vi "WSVCAP SHL FPGA TL Top Level.vi"() -> ()   [LabVIEW 2017]
uses:
  Type Defs/WSVCAP SHL State.ctl
  Type Defs/WSVCAP SHL Transaction Enum.ctl
  Type Defs/WSVCAP SHL Communication Loop State.ctl
  Type Defs/WSVCAP SHL FIFO Operation Enum.ctl
  Type Defs/WSVCAP SHL Operation Step Enum.ctl
  Type Defs/WSVCAP SHL Procedure Step Enum.ctl
  Type Defs/WSVCAP SHL Transaction Step Enum.ctl
  user.lib/Utilities/Type Defs/MISC IO Choice Enum.ctl
  <vilib>/Platform/TimedLoop/XDataNode/timing_clust.ctl
  <vilib>/Platform/TimedLoop/XDataNode/nitl_modes.ctl
  <vilib>/Platform/TimedLoop/XDataNode/wakeup.ctl
  <vilib>/rvi/Emulation/niFpgaGetClockAttributes.vi
  <vilib>/rvi/Emulation/niFpgaSctlEmulationGetInTimedLoop.vi
  <vilib>/rvi/Emulation/niFpgaEmulationReportErrorSimple.vi
  <vilib>/rvi/Emulation/niFpgaProcessEmulError.vi
  <vilib>/rvi/Emulation/niFpgaCriticalErrorInLSC.vi
  <vilib>/Platform/TimedLoop/XDataNode/XDataNode.xnode
  WSVCAP Shell FPGA Low Level/WSVCAP SHL FPGA LL I2C Debug Global.vi
  <vilib>/Platform/TimedLoop/XDataNode/XDNodeRunTimeDep.lvlib
  WSVCAP Shell FPGA Low Level/WSVCAP SHL FPGA LL RFFE Debug Global.vi
  WSVCAP Shell FPGA Low Level/FPGA-SRL/FPGA-SRL.lvlib
  WSVCAP Shell FPGA Low Level/FPGA-SRL/Debug Global.vi
panel:
  in  "UUT Set":u8=8
  in  "Stop Cycle":bool
  out "Cycle Count":u64
  in  "Socket Mask":u32=1 format="%06x"
  out "Display CH (1-48)":i32=1 min=1 max=48 step=1
  out "Status":i32
  out "Read Data":u64
  in  "Transaction":T1
  in  "Bytes to Write":u8=8
  in  "Sub Address":u8=1 format="%02x"
  in  "Ack Read Status":bool
  out "Read Status Flag":bool
  in  "Exit":bool
  out "Waveform Chart":cluster{i16, i16, i16, i16}(graph)
  in  "Wait Ticks":u32=20
  in  "Slave Address":u8=1 format="%02x"
  in  "Bytes to Read":u8=8
  in  "Start":bool
  in  "Cmd":T2
  in  "Ack Read":bool
  out "Read Flag":bool
  in  "Write Flag":bool
  in  "Write Data":u64
  # "Control"
  # "Configuration Parameters"
  # "Host Data Transfer"
  # "Command Type"
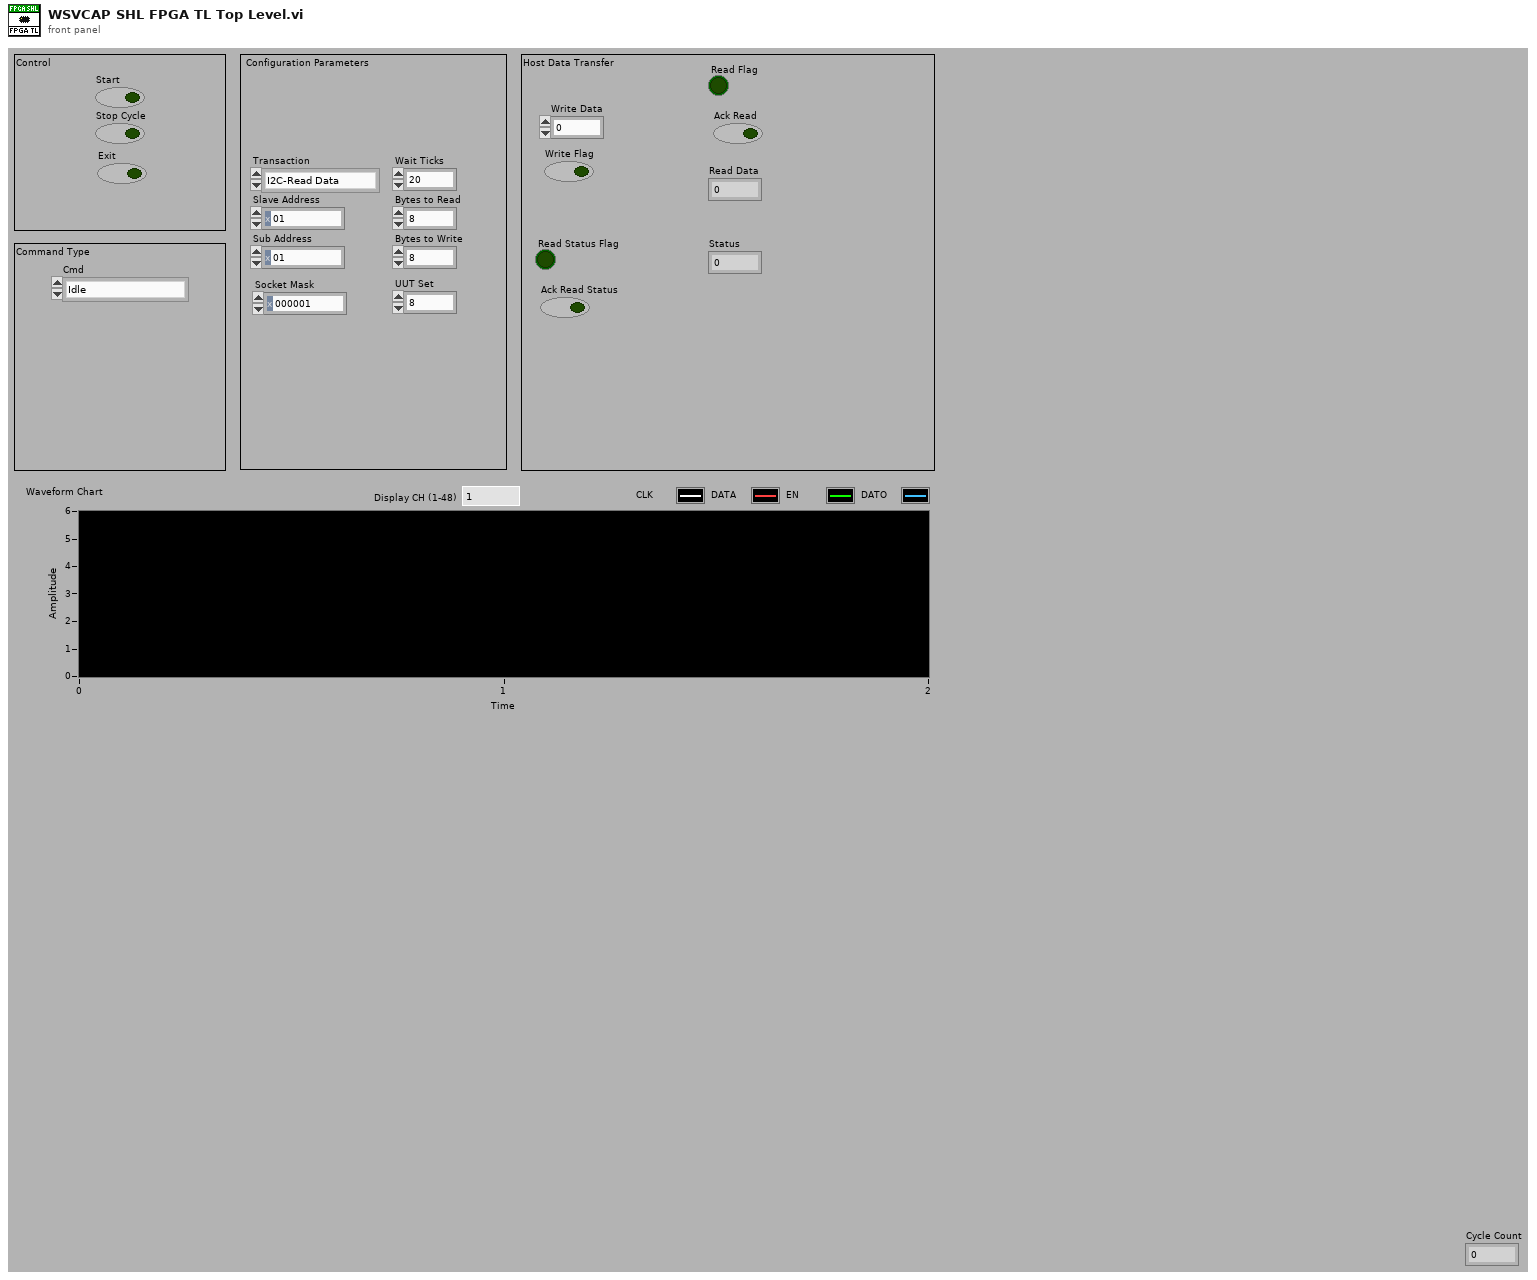
[diagram p1: front panel]
types:
  T1 = typedef "WSVCAP SHL Transaction Enum.ctl" = enum16{"I2C-Read Data", "I2C-Write Data", "RFFE-Ext Write", "RFFE-Ext Read", "SRL-Write Data"}
  T2 = typedef "WSVCAP SHL State.ctl" = enum8{"Idle", "Transfer Data"}
  T3 = typedef "WSVCAP SHL Communication Loop State.ctl" = enum8{"Idle", "Initialize", "Pre-Transmission", "Transmit Data", "Post Transmition", "Operation Complete"}
  T4 = typedef "WSVCAP SHL FIFO Operation Enum.ctl" = enum16{"Create FIFO/Memory", "Get Write FIFO Status", "Get Read FIFO Status", "Put Element in Write", "Put Element in Read", "Get Element from Write", "Get Element from Read"}
  T5 = typedef "WSVCAP SHL Procedure Step Enum.ctl" = enum16{"I2C Start/Stop - 1: Set Clock Low", "I2C Start/Stop - 2: Wait", "I2C Start/Stop - 3: Set Data I", "I2C Start/Stop - 4: Wait", "I2C Start/Stop - 5: Set Clock High", "I2C Start/Stop - 6: Wait", "I2C Start/Stop - 7: Set Data II", "I2C Start/Stop - 8: Wait", "I2C Start/Stop - 9: Set Clock Low", "I2C Start/Stop - 10: Wait", "I2C Read ACK - 1: Set Clock High", "I2C Read ACK - 2: Wait", "I2C Read ACK - 3: Read ACK Bit", "I2C Read ACK - 4: Wait", "I2C Read ACK - 5: Set Clock Low", "I2C Read ACK - 6: Wait", "I2C Write ACK - 1: Write ACK Bit", "I2C Write ACK - 2: Wait", "I2C Write ACK - 3: Set Clock High", "I2C Write ACK - 4: Wait", "I2C Write ACK - 5: Set Clock Low", "I2C Write ACK - 6: Wait", "I2C Write ACK - 7: Set Data Low", "I2C Send Add - 1: Reset Bits Remaining", "I2C Send Add - 2: Set Data Bit", "I2C Send Add - 3: Wait", "I2C Send Add - 4: Set Clock High", "I2C Send Add - 5: Wait", "I2C Send Add - 6: Set Clock Low", "I2C Send Add - 7: Wait", "I2C Send Add - 8: Check Bits Remaining", "I2C Send Data - 1: Reset Bits Remaining", "I2C Send Data - 2: Load Write Bit from FIFO", "I2C Send Data - 3: Set Data Bit", "I2C Send Data - 4: Wait", "I2C Send Data - 5: Set Clock High", "I2C Send Data - 6: Wait", "I2C Send Data - 7: Set Clock Low", "I2C Send Data - 8: Wait", "I2C Send Data - 9: Check Bits Remaining", "I2C Receive Data - 1: Reset Bits Remaining", "I2C Receive Data - 2: Wait", "I2C Receive Data - 3: Set Clock High", "I2C Receive Data - 4: Wait", "I2C Receive Data - 5: Read Data Bit", "I2C Receive Data - 6: Wait", "I2C Receive Data - 7: Set Clock Low", "I2C Receive Data - 8: Wait", "I2C Receive Data - 9: Check Bits Remaining", "RFFE Send SSC - 1:Set Low", "RFFE Send SSC - 2:Wait", "RFFE Send SSC - 3:Set SDA High", "RFFE Send SSC - 4:Wait", "RFFE Send SSC - 5:Set SDA Low", "RFFE Send SSC - 6:Wait", "RFFE Send Data - 1:Set SCL High", "RFFE Send Data - 2:Wait", "RFFE Send Data - 3:Set SCL Low", "RFFE Send Data - 4:Wait", "RFFE Send Data - 5:Set SCL High (P)", "RFFE Send Data - 6:Wait", "RFFE Send Data - 7:Set SCL Low (P)", "RFFE Send Data - 8:Wait", "RFFE Send Data - 9:Set SCL High (BP)", "RFFE Send Data - 10:Wait", "RFFE Send Data - 11:Set SCL Low (BP)", "RFFE Send Data - 12:Wait", "RFFE Receive Data - 1:Set SCL High", "RFFE Receive Data - 2:Wait", "RFFE Receive Data - 3:Set SCL Low", "RFFE Receive Data - 4:Wait", "RFFE Receive Data - 5:Set SCL High (BP)", "RFFE Receive Data - 6:Wait", "RFFE Receive Data - 7:Set SCL Low (BP)", "RFFE Receive Data - 8:Wait", "RFFE Wait CMD Delay - 1:Wait", "RFFE Clear Lines - 1:Clear", "SRL Write Data - 1:Set SYNC High", "SRL Write Data - 2:Wait SYNC Delay", "SRL Write Data - 3:Set SYNC Low", "SRL Write Data - 4:Set SCLK High", "SRL Write Data - 5:Wait", "SRL Write Data - 6:Set SCLK Low", "SRL Write Data - 7:Wait", "SRL Write Data - 8:Set SYNC High", "SRL Wait CMD Delay - 1:Wait", "SRL Clear Lines - 1:Clear"}
  T6 = typedef "WSVCAP SHL Operation Step Enum.ctl" = enum16{"I2C Send Slave Add - A: Send Start Sequence", "I2C Send Slave Add - B: Load Address Byte", "I2C Send Slave Add - C: Send Address Byte", "I2C Send Slave Add - D: Read Slave ACK", "I2C Send Sub Add - A: Load Sub Address", "I2C Send Sub Add - B: Send Address Byte", "I2C Send Sub Add - C: Read Slave ACK", "I2C Send Data - A: Get Byte from FIFO", "I2C Send Data - B: Send Data Byte", "I2C Send Data - C: Read Slave ACK", "I2C Send Data - D: Send Stop Sequence", "I2C Read Data - A: Load Bytes to Read", "I2C Read Data - B: Receive Byte", "I2C Read Data - C: Write Master ACK", "I2C Read Data - D: Send Stop Sequence", "RFFE Read Data - A: Send SSC", "RFFE Read Data - B: Send CMD Frame", "RFFE Read Data - C: Receive Byte", "RFFE Write Data - A: Send SSC", "RFFE Write Data - B: Send Data", "RFFE Write Data - C: Wait CMD Delay", "RFFE Write Data - D: Clear Lines", "SRL Write Data - A: Send Data", "SRL Write Data - B: Wait CMD Delay", "SRL Write Data - C: Clear Lines"}
  T7 = typedef "WSVCAP SHL Transaction Step Enum.ctl" = enum16{"I2C Write - I:Send Slave Address", "I2C Write - II:Send Sub Address", "I2C Write - III:Send Data Bytes", "I2C Read - I:Send Slave Address (W)", "I2C Read - II:Send Sub Address", "I2C Read - III:Send Slave Address (R)", "I2C Read - IV:Read Data Bytes", "RFFE Ext Write - I.Write Data", "RFFE Ext Read - I:Read Data", "SRL Write - I:Write Data"}
  T8 = typedef "MISC IO Choice Enum.ctl" = enum16{"Read", "Write"}
  T9 = typedef "XDNodeRunTimeDep.lvlib/timing_clust.ctl" = cluster{"Expected End [f-1]":u64, "Actual End [f-1]":u64, "Finished Late? [f-1]":bool, "Expected End [i-1]":u64, "Actual End [i-1]":u64, "Finished Late? [i-1]":bool, "Expected Start [i]":u64, "Actual Start [i]":u64, "Expected Start [f]":u64, "Actual Start [f]":u64, "Source Name":string, "Structure Name":string, "Period":i64, "Deadline":i64, "Offset":i64, "Start":i64, "Priority":i32, "Timeout":i32, "Mode":T10, "Wakeup Reason":T11, "Error":errorcluster, "Source Type":string, "Secondary Source Type":string, "Global End Time":u64, "Global Start Time":u64, "Frame Duration":u64, "Iteration Duration":u64, "Assigned CPU":i32, "I/O Scan Engine Mode":u32}
  T10 = typedef "XDNodeRunTimeDep.lvlib/nitl_modes.ctl" = enum32{"No Change", "Process missed periods, maintain original phase", "Discard missed periods, maintain original phase", "Process missed periods, ignore original phase", "Discard missed periods, ignore original phase"}
  T11 = typedef "XDNodeRunTimeDep.lvlib/wakeup.ctl" = enum32{"Normal", "Aborted", "Asynchronous wakeup", "Timing source error", "Timed loop error", "Timeout"}
  T12 = typedef "WSVCAP SHL Transaction Cluster.ctl" = cluster{"Transaction":T1, "Write Byte":u8, "Write Bits Remaining":u8, "Read Bits Remaining":u8, "Read Bytes Remaining":u8, "Wait Ticks Remaining":u32, "Slave Address":u8, "Bytes to Read":u8, "Bytes to Write":u8, "Sub Address":u8, "Socket Mask":u32, "Write CMD Idx [0-95]":u8, "Write Bit Index [0-18]":u8, "CMD Delay (Ticks)":u32, "Commands per Cycle [1-96]":u8, "CMD Length [1-48]":u8, "Cycle Count":u64, "Cycle Mode":bool, "Cycle CMD":u64, "Transaction Step":T7, "Operation Step":T6, "Procedure Step":T5, "Start Operation":bool, "Start Procedure":bool, "Procedure":T13, "Wait Ticks":u32, "UUT Set (0/1)":u8}
  T13 = typedef "WSVCAP SHL Procedure Enum.ctl" = enum16{"None", "I2C-Send Start/Stop Sequence", "I2C-Send Address Byte", "I2C-Send Data Byte", "I2C-Read ACK", "I2C-Receive Byte", "I2C-Write ACK", "RFFE-Clear Lines", "RFFE-Send SSC", "RFFE-Send Data", "RFFE-Receive Data", "RFFE-Wait CMD Delay", "SRL-Clear Lines", "SRL-Send Data", "SRL-Wait CMD Delay"}
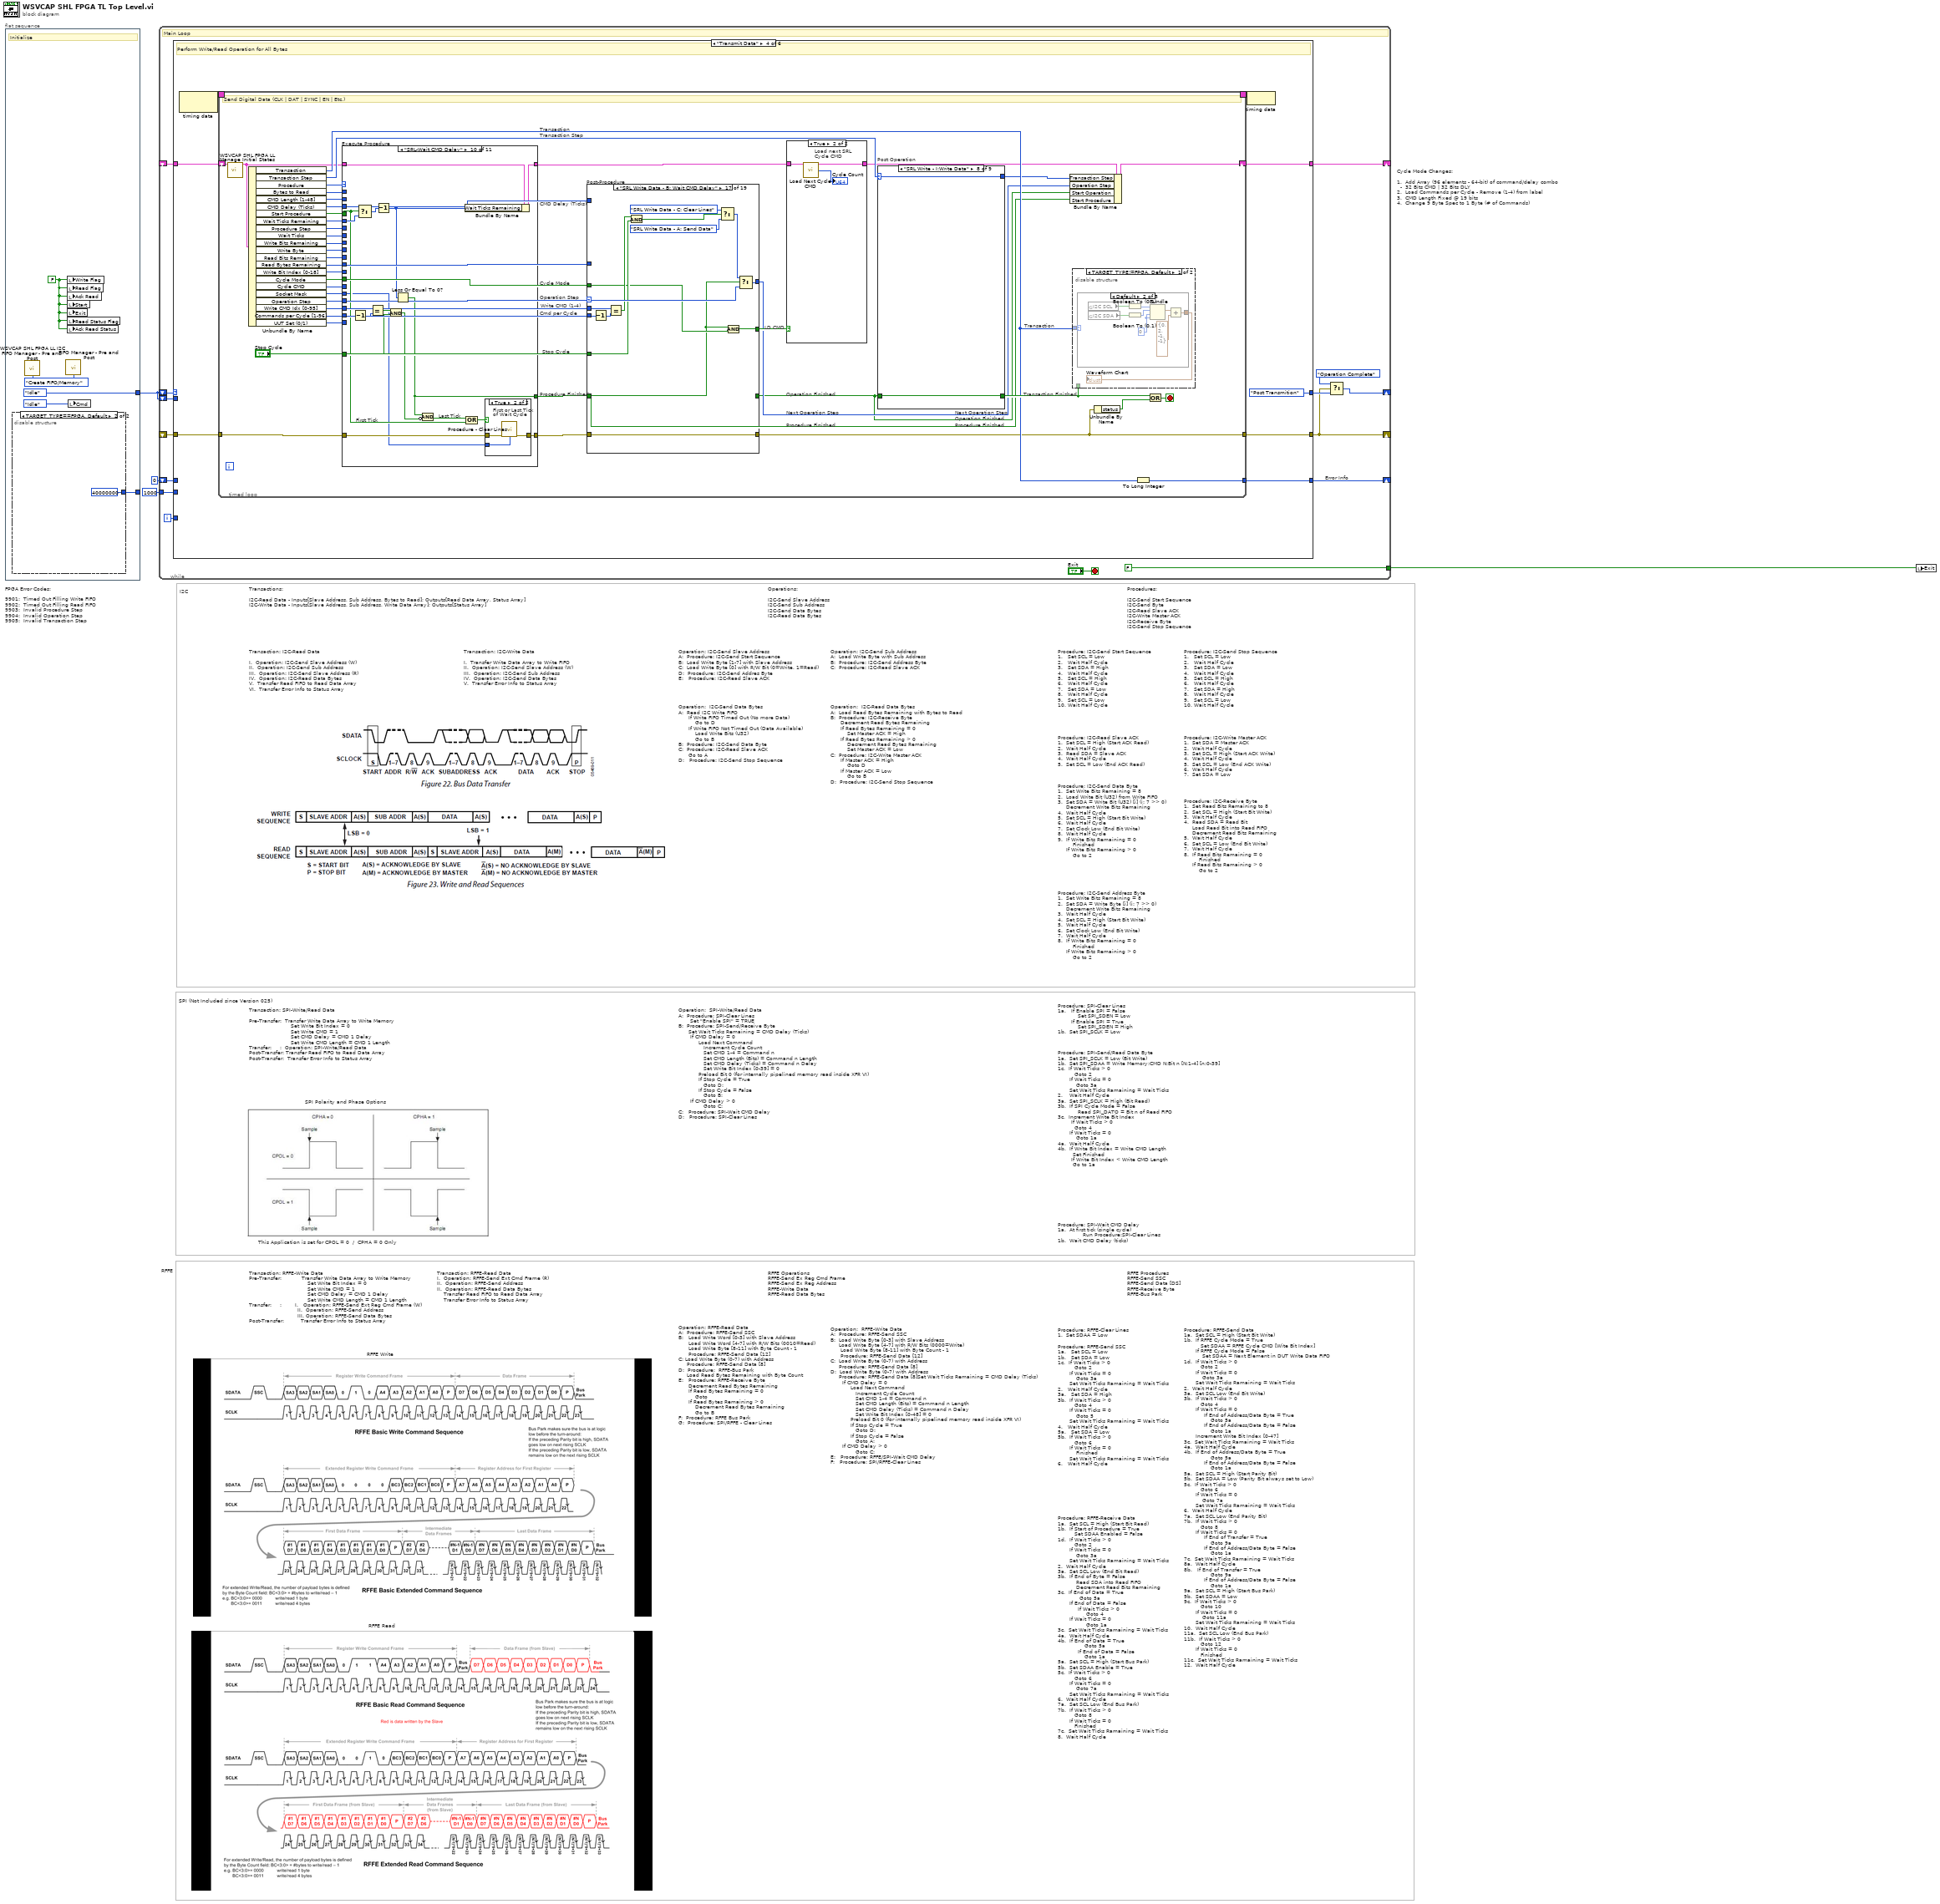
[diagram p0: block diagram]
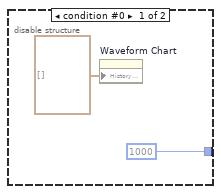
[diagram p2: hidden frame]
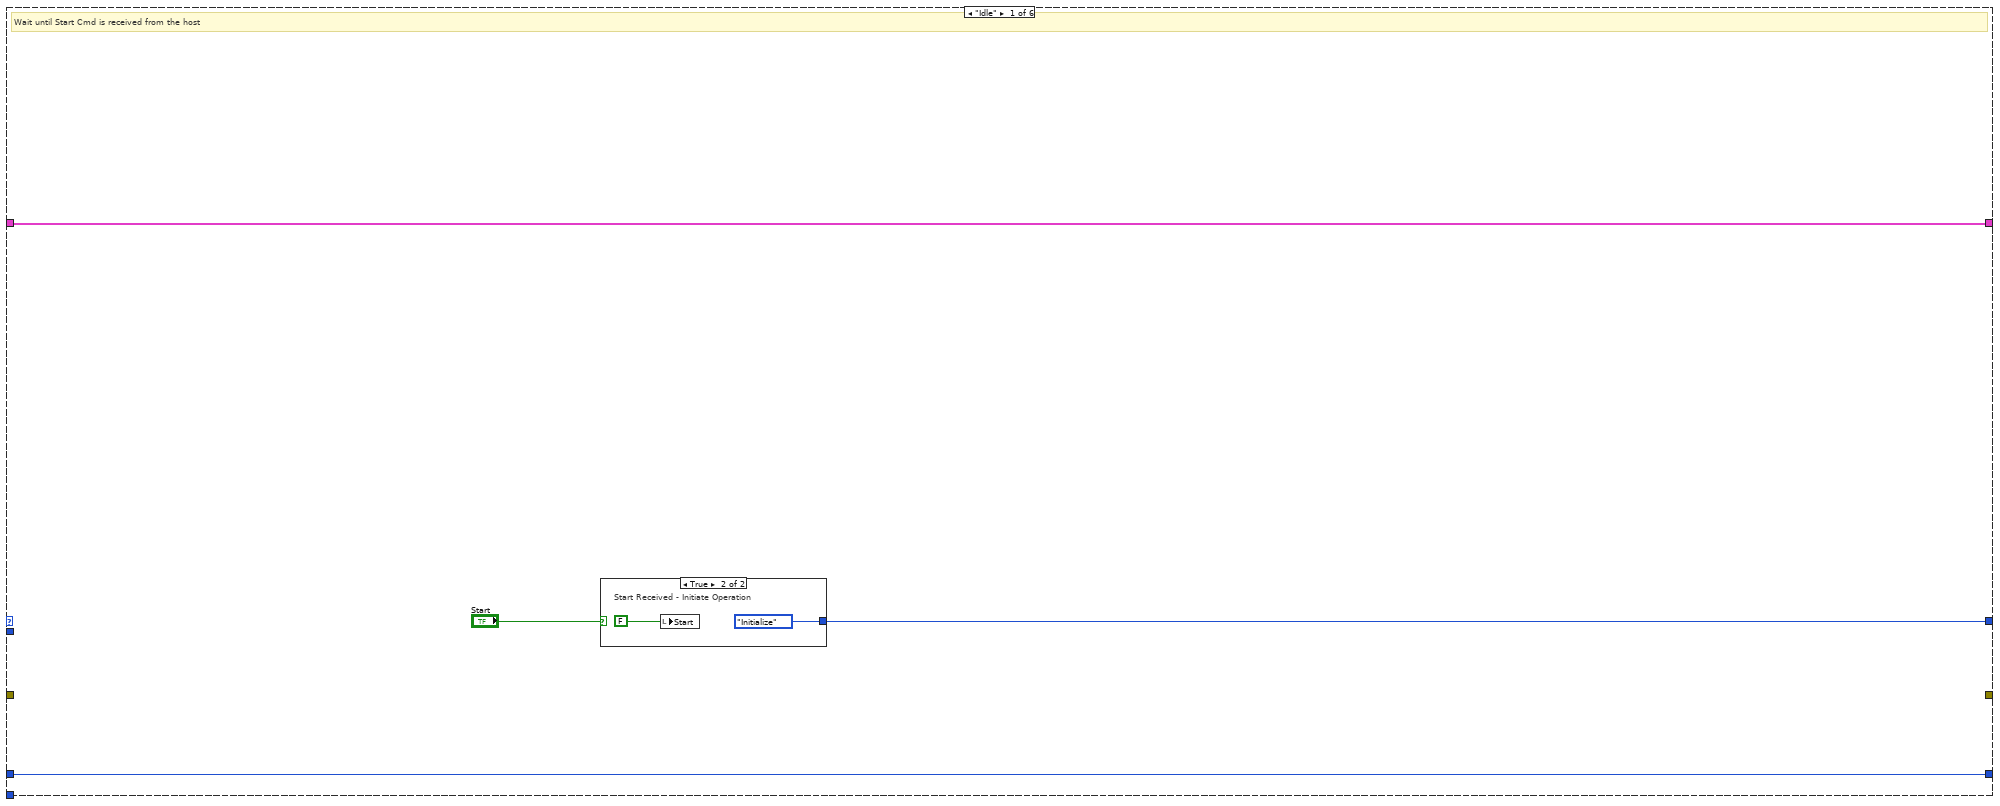
[diagram p3: hidden frame]
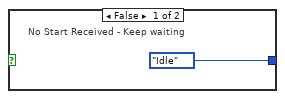
[diagram p4: hidden frame]
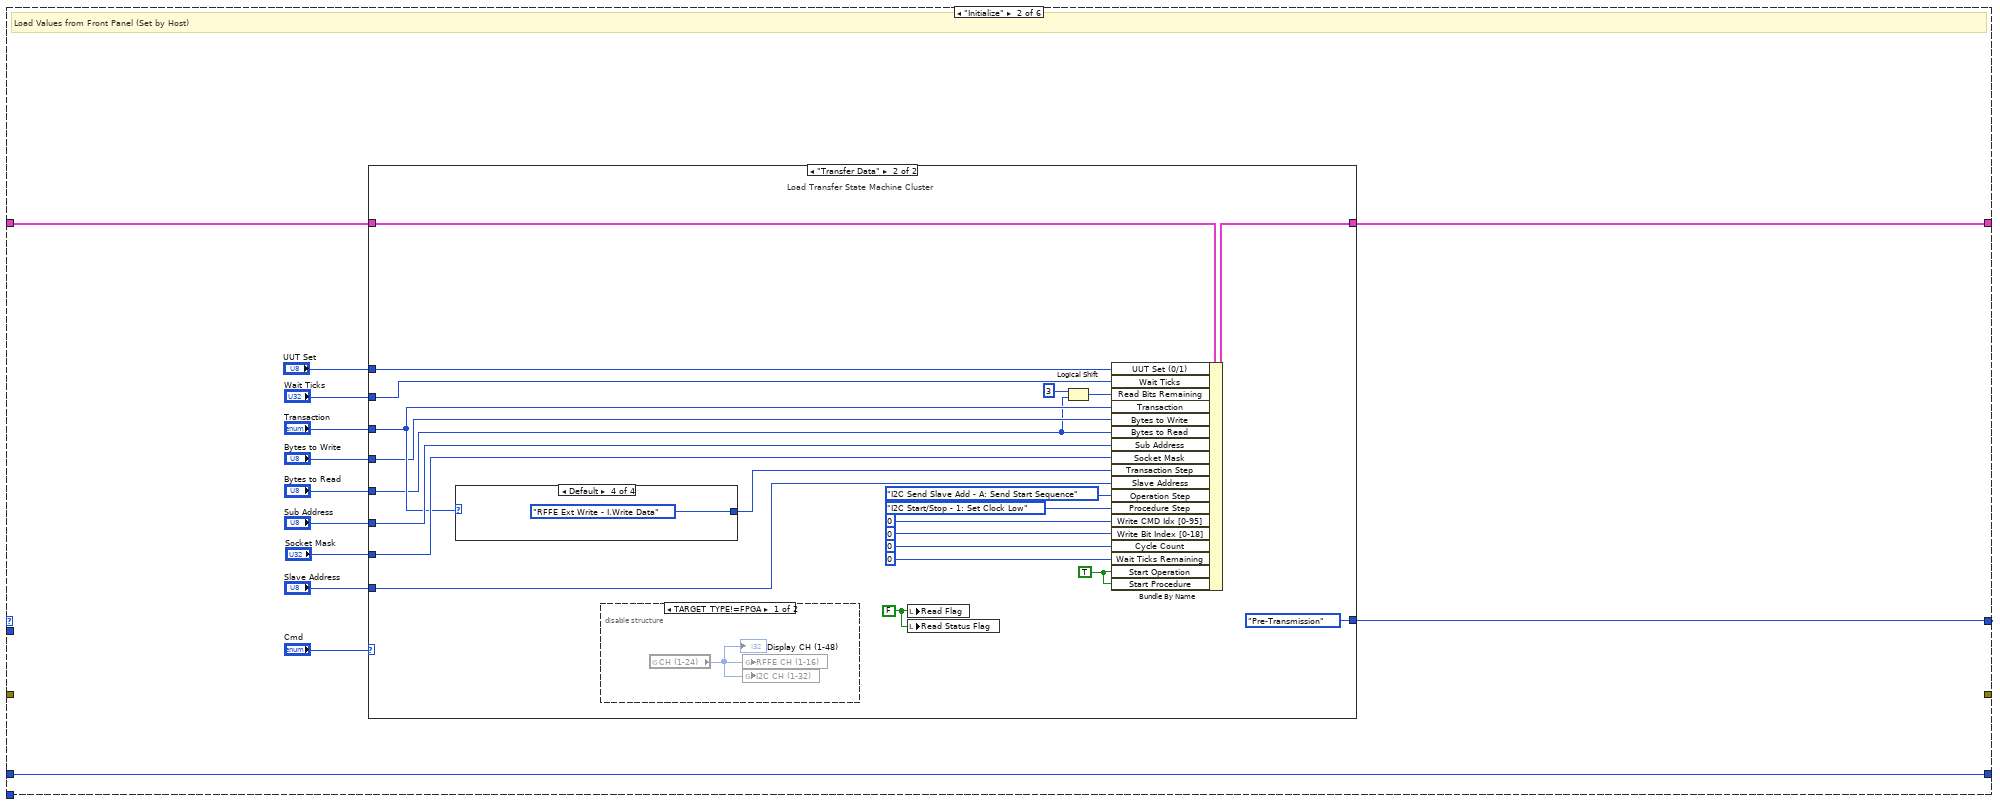
[diagram p5: hidden frame]
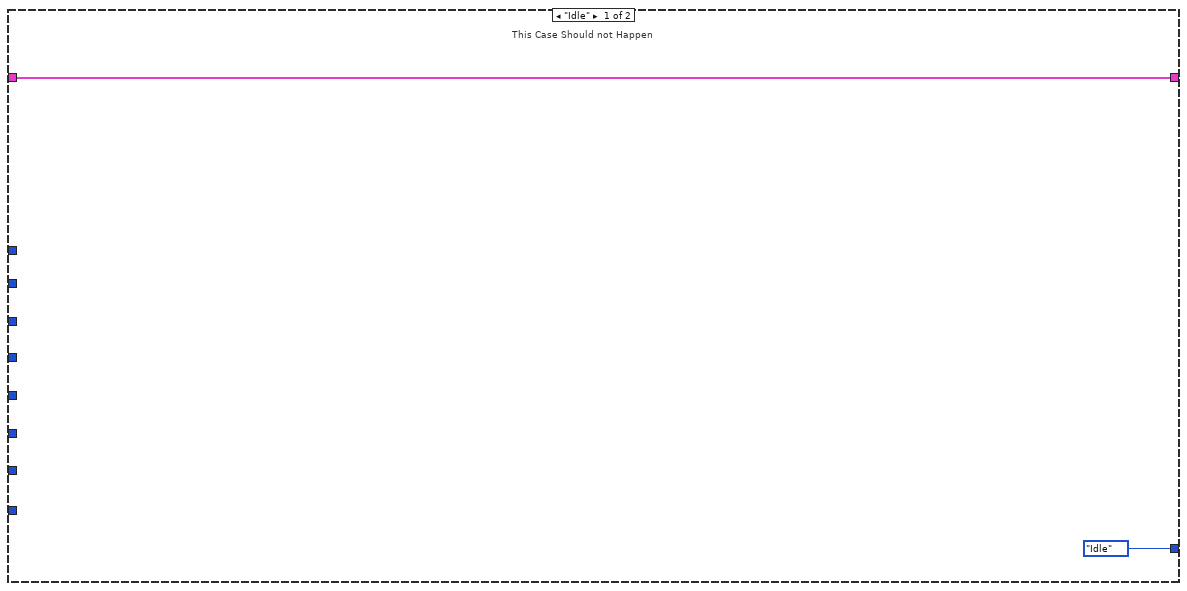
[diagram p6: hidden frame]
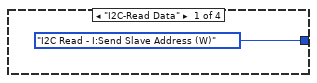
[diagram p7: hidden frame]
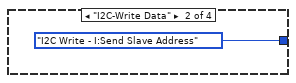
[diagram p8: hidden frame]
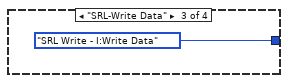
[diagram p9: hidden frame]
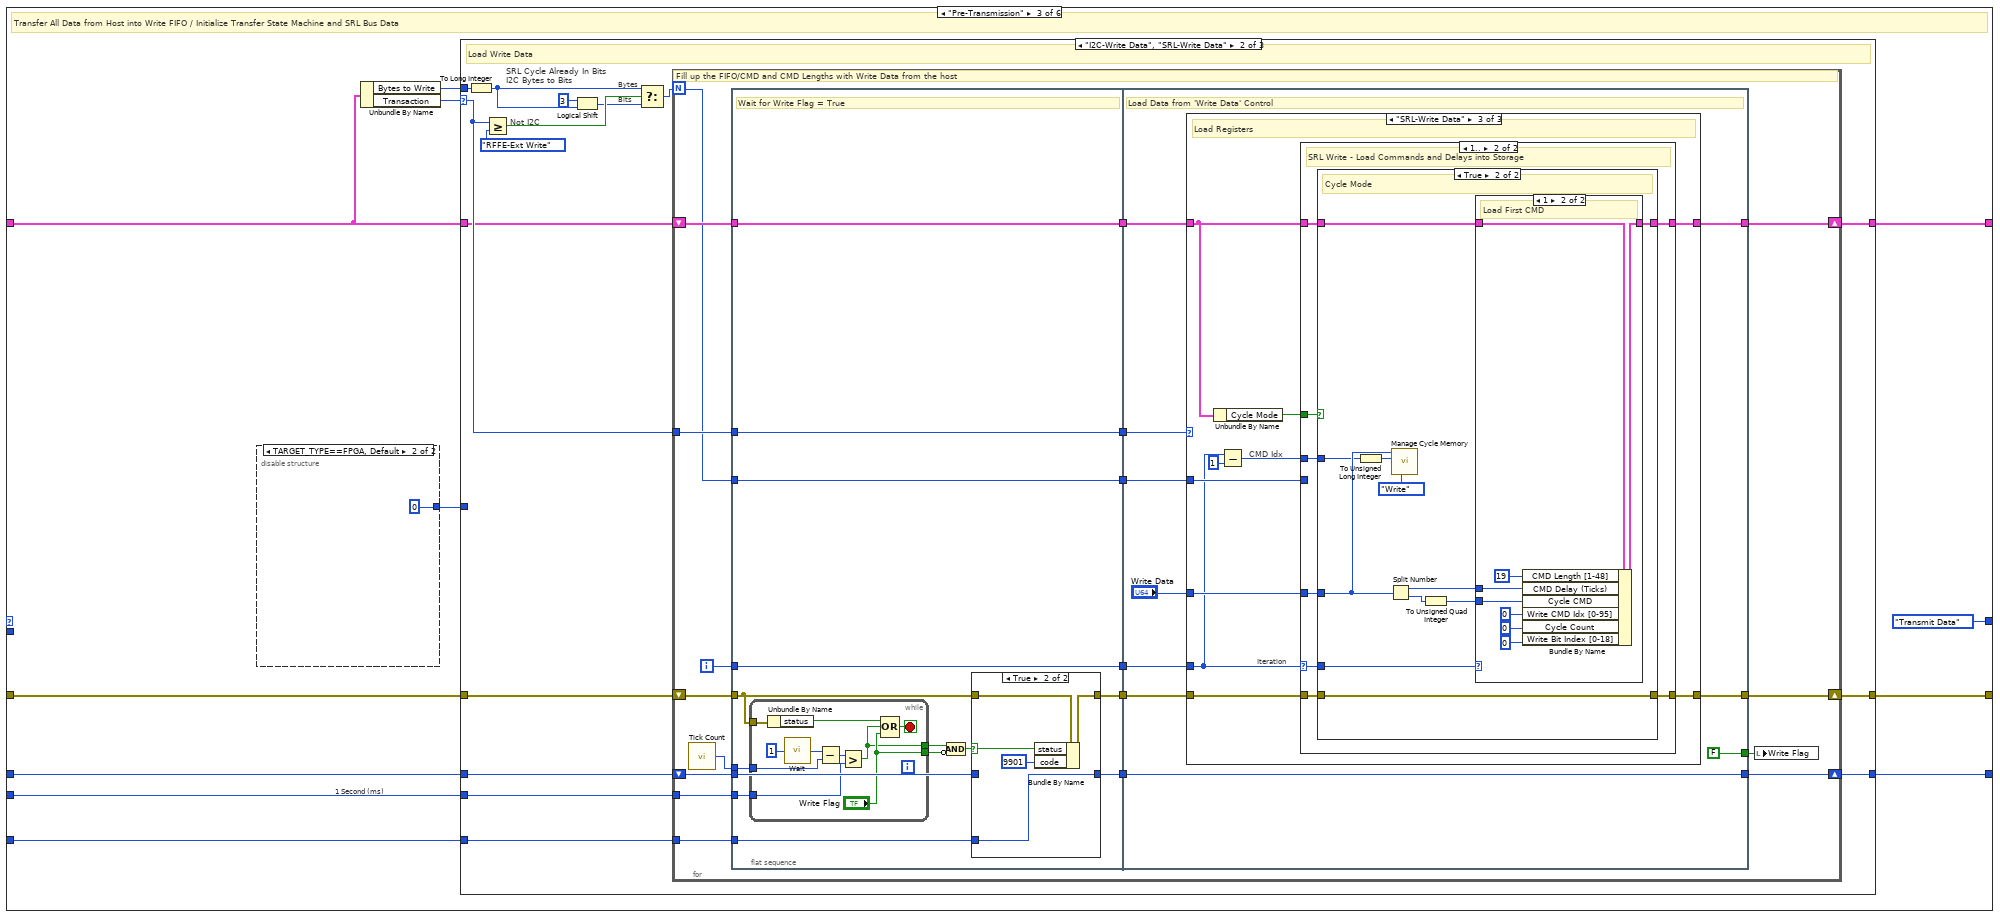
[diagram p11: hidden frame]
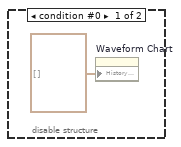
[diagram p12: hidden frame]
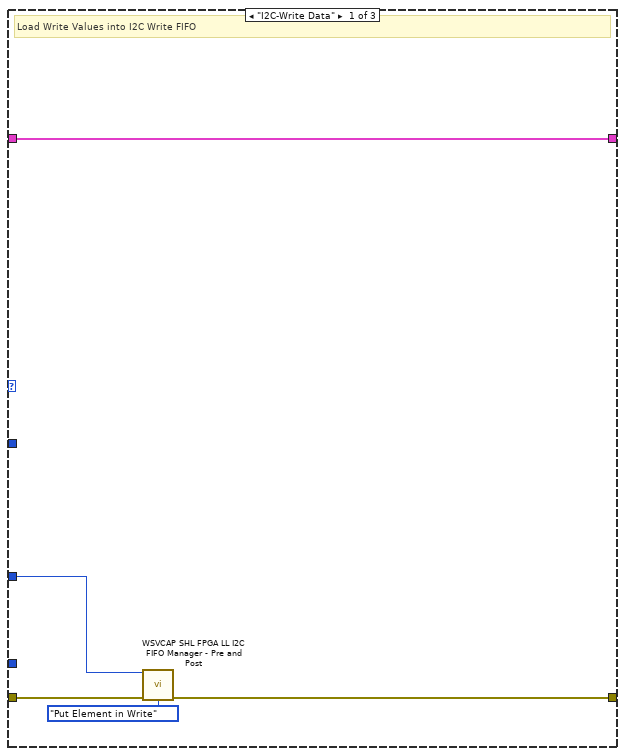
[diagram p15: hidden frame]
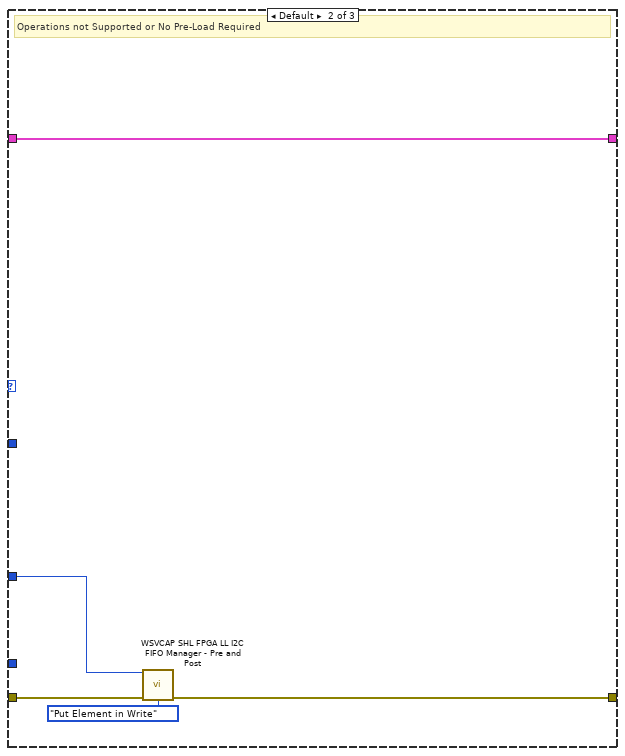
[diagram p16: hidden frame]
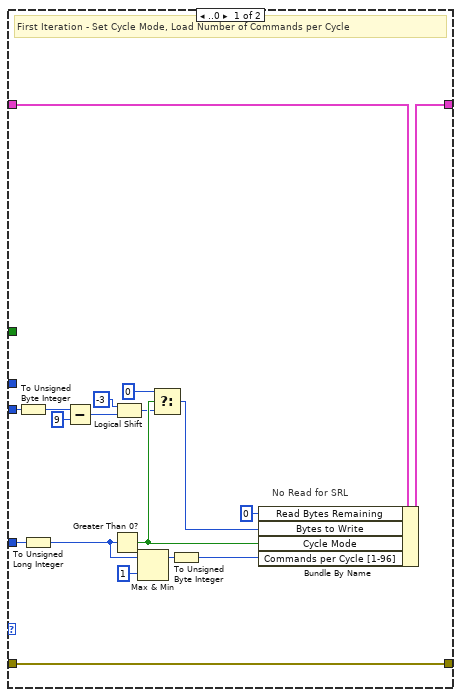
[diagram p17: hidden frame]
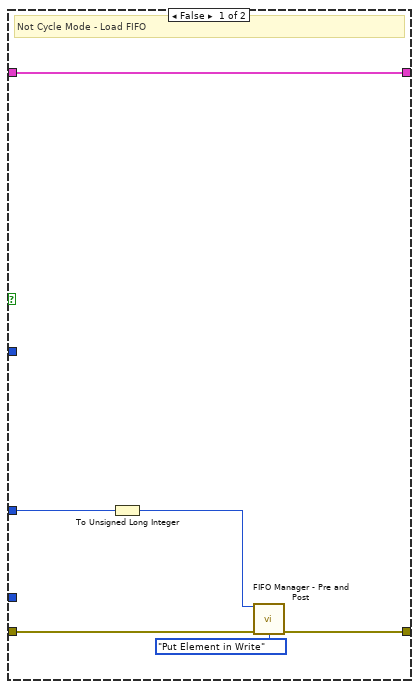
[diagram p18: hidden frame]
diagram:
  # "Cycle Mode Changes:\n\n1.  Add Array (96 elements - 64-bit) of command/delay combo\n  -  32 Bits CMD | 32 Bits DLY\n2.  Load Commands per Cycle - Remove (1-4) from label\n3.  CMD Length Fixed @ 19 bits\n4.  Change 9 Byte Spec to 1 Byte (# of Commands)"
  # "RFFE"
  # "SPI (Not Included since Version 025)"
  # "I2C"
  # "Procedure: RFFE-Receive Data\n1a.  Set SCL = High (Start Bit Read)\n1b.  If Start of Procedure = True\n          Set SDAA Enabled = False\n1d.  If Wait Ticks > 0\n          Goto 2\n       If Wait Ticks = 0 \n           Goto 3a\n       Set Wait Ticks Ramaining = Wait Ticks\n2.  Wait Half Cycle\n3a.  Set SCL Low (End Bit Read)\n3b.  If End of Byte = False\n           Read SDA into Read FIFO\n           Decrement Read Bits Remaining\n3c.  If End of Data = True\n             Goto 5a\n       If End of Data = False\n            If Wait Ticks > 0\n                 Goto 4\n       If Wait Ticks = 0         \n                 Goto 1a\n3c.  Set Wait Ticks Ramaining = Wait Ticks     \n4a.  Wait Half Cycle\n4b.  If End of Data = True\n                Goto 5a\n            If End of Data = False\n                Goto 1a\n5a.  Set SCL = High (Start Bus Park)\n5b.  Set SDAA Enable = True\n5c.  If Wait Ticks > 0\n          Goto 6\n       If Wait Ticks = 0 \n           Goto 7a\n       Set Wait Ticks Ramaining = Wait Ticks\n6.  Wait Half Cycle\n7a.  Set SCL Low (End Bus Park)\n7b.  If Wait Ticks > 0\n          Goto 8\n       If Wait Ticks = 0 \n          Finished\n7c.  Set Wait Ticks Ramaining = Wait Ticks\n8.  Wait Half Cycle"
  # "Procedure: RFFE-Send Data\n1a.  Set SCL = High (Start Bit Write)\n1b.  If RFFE Cycle Mode = True\n          Set SDAA = RFFE Cycle CMD [Wite Bit Index]\n       If RFFE Cycle Mode = False\n           Set SDAA = Next Element in DUT Write Data FIFO\n1d.  If Wait Ticks > 0\n          Goto 2\n       If Wait Ticks = 0 \n           Goto 3a\n       Set Wait Ticks Ramaining = Wait Ticks\n2.  Wait Half Cycle\n3a.  Set SCL Low (End Bit Write)\n3b.  If Wait Ticks > 0\n          Goto 4\n       If Wait Ticks = 0 \n            If End of Address/Data Byte = True\n                Goto 5a\n            If End of Address/Data Byte = False\n                Goto 1a\n       Increment Write Bit Index [0-47]\n3c.  Set Wait Ticks Ramaining = Wait Ticks     \n4a.  Wait Half Cycle\n4b.  If End of Address/Data Byte = True\n                Goto 5a\n            If End of Address/Data Byte = False\n                Goto 1a\n5a.  Set SCL = High (Start Parity Bit)\n5b.  Set SDAA = Low (Parity Bit always set to Low)\n5c.  If Wait Ticks > 0\n          Goto 6\n       If Wait Ticks = 0 \n           Goto 7a\n       Set Wait Ticks Ramaining = Wait Ticks\n6.  Wait Half Cycle\n7a.  Set SCL Low (End Parity Bit)\n7b.  If Wait Ticks > 0\n          Goto 8\n       If Wait Ticks = 0 \n            If End of Transfer = True\n                Goto 9a\n            If End of Address/Data Byte = False\n                Goto 1a\n7c.  Set Wait Ticks Ramaining = Wait Ticks\n8a.  Wait Half Cycle\n8b.   If End of Transfer = True\n                Goto 9a\n            If End of Address/Data Byte = False\n                Goto 1a\n9a.  Set SCL = High (Start Bus Park)\n9b.  Set SDAA = Low\n9c.  If Wait Ticks > 0\n          Goto 10\n       If Wait Ticks = 0 \n           Goto 11a\n       Set Wait Ticks Ramaining = Wait Ticks\n10.  Wait Half Cycle\n11a.  Set SCL Low (End Bus Park)\n11b.  If Wait Ticks > 0\n          Goto 12\n       If Wait Ticks = 0 \n          Finished\n11c.  Set Wait Ticks Ramaining = Wait Ticks\n12.  Wait Half Cycle"
  # "Procedure: RFFE-Send SSC\n1a.   Set SCL = Low\n1b.   Set SDA = Low\n1c.  If Wait Ticks > 0\n          Goto 2\n       If Wait Ticks = 0 \n           Goto 3a\n       Set Wait Ticks Ramaining = Wait Ticks\n2.   Wait Half Cycle\n3a.   Set SDA = High\n3b.  If Wait Ticks > 0\n          Goto 4\n       If Wait Ticks = 0 \n           Goto 5\n       Set Wait Ticks Ramaining = Wait Ticks\n4.   Wait Half Cycle\n5a.   Set SDA = Low\n5b.  If Wait Ticks > 0\n          Goto 6\n       If Wait Ticks = 0 \n           Finished\n       Set Wait Ticks Ramaining = Wait Ticks\n6.   Wait Half Cycle"
  # "Procedure: SPI-Clear Lines\n1a.   If Enable SPI = False\n            Set SPI_SDEN = Low\n        If Enable SPI = True\n            Set SPI_SDEN = High\n1b.  Set SPI_SCLK = Low"
  # "Procedure: RFFE-Clear Lines\n1.  Set SDAA = Low"
  # "Operation:  RFFE-Write Data\nA:  Procedure: RFFE-Send SSC\nB:  Load Write Byte [0-3] with Slave Address\n     Load Write Byte [4-7] with R/W Bits (0000=Write)\n      Load Write Byte [8-11] with Byte Count - 1\n      Procedure: RFFE-Send Data [12]\nC:  Load Write Byte (0-7) with Address\n     Procedure: RFFE-Send Data [8]\nD:  Load Write Byte (0-7) with Address\n     Procedure: RFFE-Send Data [8]Set Wait Ticks Remaining = CMD Delay (Ticks)\n       If CMD Delay = 0\n            Load Next Command\n               Increment Cycle Count\n               Set CMD 1-4 = Command n\n               Set CMD Length (Bits) = Command n Length\n               Set CMD Delay (Ticks) = Command n Delay\n               Set Write Bit Index [0-48] = 0\n            Preload Bit 0 (for internally pipelined memory read inside XFR VI)\n            If Stop Cycle = True\n               Goto D:\n            If Stop Cycle = False\n               Goto A:\n       If CMD Delay > 0\n               Goto C:\nE:   Procedure: RFFE/SPI-Wait CMD Delay          \nF:   Procedure: SPI/RFFE-Clear Lines"
  # "Operation: RFFE-Read Data\nA:  Procedure: RFFE-Send SSC\nB:   Load Write Word [0-3] with Slave Address\n      Load Write Word [4-7] with R/W Bits (0010=Read)\n      Load Write Byte [8-11] with Byte Count - 1\n      Procedure: RFFE-Send Data [12]\nC: Load Write Byte (0-7) with Address\n     Procedure: RFFE-Send Data [8]\nD:  Procedure:  RFFE-Bus Park\n     Load Read Bytes Remaining with Byte Count\nE:   Procedure: RFFE-Receive Byte\n      Decrement Read Bytes Remaining\n      If Read Bytes Remaining = 0\n          Goto\n      If Read Bytes Remaining > 0\n          Decrement Read Bytes Remaining\n          Go to B\nF:  Procedure: RFFE Bus Park\nG:  Procedure: SPI/RFFE - Clear Lines"
  # "RFFE Write"
  # "RFFE Read"
  # "Transaction: RFFE-Write Data\nPre-Transfer:            Transfer Write Data Array to Write Memory\n                                   Set Write Bit Index = 0\n                                   Set Write CMD = 1\n                                   Set CMD Delay = CMD 1 Delay\n                                   Set Write CMD Length = CMD 1 Length\nTransfer:     :        I.   Operation: RFFE-Send Ext Reg Cmd Frame (W)\n                             II.  Operation: RFFE-Send Address\n                             III. Operation: RFFE-Send Data Bytes\nPost-Transfer:          Transfer Error Info to Status Array"
  # "RFFE Procedures\nRFFE-Send SSC\nRFFE-Send Data [DS]\nRFFE-Receive Byte\nRFFE-Bus Park"
  # "Transaction: RFFE-Read Data\nI.  Operation: RFFE-Send Ext Cmd Frame (R)\nII.  Operation: RFFE-Send Address\nII.  Operation: RFFE-Read Data Bytes\n    Transfer Read FIFO to Read Data Array\n    Transfer Error Info to Status Array"
  # "RFFE Operations\nRFFE-Send Ex Reg Cmd Frame\nRFFE-Send Ex Reg Address\nRFFE-Write Data\nRFFE-Read Data Bytes"
  # "SPI Polarity and Phase Options"
  # "Procedure: SPI-Wait CMD Delay\n1a.  At first tick (single cycle)\n               Run Procedure:SPI-Clear Lines\n1b.  Wait CMD Delay (ticks)"
  # "This Application is set for CPOL = 0  /  CPHA = 0 Only"
  # "Procedure: SPI-Send/Read Data Byte\n1a.  Set SPI_SCLK = Low (Bit Write)\n1b.  Set SPI_SDAA = Write Memory:CMD N:Bit n [N:1-4] [n:0-39] \n1c.  If Wait Ticks > 0\n          Goto 2\n       If Wait Ticks = 0 \n           Goto 3a\n       Set Wait Ticks Ramaining = Wait Ticks\n2.    Wait Half Cycle\n3a.  Set SPI_SCLK = High (Bit Read)\n3b.  If SPI Cycle Mode = False\n            Read SPI_DATO = Bit n of Read FIFO            \n3c.  Increment Write Bit Index\n        If Wait Ticks > 0\n          Goto 4\n       If Wait Ticks = 0 \n           Goto 1a \n4a.  Wait Half Cycle\n4b.  If Write Bit Index = Write CMD Length\n         Set Finished\n        If Write Bit Index < Write CMD Length\n         Go to 1a"
  # "Operation:  SPI-Write/Read Data\nA:  Procedure: SPI-Clear Lines\n       Set \"Enable SPI\" = TRUE \nB:  Procedure: SPI-Send/Receive Byte\n      Set Wait Ticks Remaining = CMD Delay (Ticks)\n       If CMD Delay = 0\n            Load Next Command\n               Increment Cycle Count\n               Set CMD 1-4 = Command n\n               Set CMD Length (Bits) = Command n Length\n               Set CMD Delay (Ticks) = Command n Delay\n               Set Write Bit Index [0-39] = 0\n            Preload Bit 0 (for internally pipelined memory read inside XFR VI)\n            If Stop Cycle = True\n               Goto D:\n            If Stop Cycle = False\n               Goto B:\n       If CMD Delay > 0\n               Goto C:\nC:   Procedure: SPI-Wait CMD Delay          \nD:   Procedure: SPI-Clear Lines"
  # "FPGA Error Codes:\n\n9901:  Timed Out Filling Write FIFO\n9902:  Timed Out Filling Read FIFO\n9903:  Invalid Procedure Step\n9904:  Invalid Operation Step\n9905:  Invalid Transaction Step"
  # "Transaction: SPI-Write/Read Data\n\nPre-Transfer:  Transfer Write Data Array to Write Memory\n                         Set Write Bit Index = 0\n                         Set Write CMD = 1\n                         Set CMD Delay = CMD 1 Delay\n                         Set Write CMD Length = CMD 1 Length\nTransfer:     :  Operation: SPI-Write/Read Data\nPost-Transfer: Transfer Read FIFO to Read Data Array\nPost-Transfer:  Transfer Error Info to Status Array"
  # "Procedure: I2C-Send Address Byte\n1.  Set Write Bits Remaining = 8\n2.  Set SDA = Write Byte [i] (i: 7 >> 0)\n     Decrement Write Bits Remaining\n3.  Wait Half Cycle\n4.  Set SCL = High (Start Bit Write)\n5.  Wait Half Cycle\n6.  Set Clock Low (End Bit Write)\n7.  Wait Half Cycle\n8.  If Write Bits Remaining = 0\n         Finished\n     If Write Bits Remaining > 0\n         Go to 2"
  # "Procedure: I2C-Write Master ACK\n1.  Set SDA = Master ACK\n2.  Wait Half Cycle\n3.  Set SCL = High (Start ACK Write)\n4.  Wait Half Cycle\n5.  Set SCL = Low (End ACK Write)\n6.  Wait Half Cycle\n7.  Set SDA = Low"
  # "Procedure: I2C-Send Start Sequence\n1.   Set SCL = Low\n2.   Wait Half Cycle\n3.   Set SDA = High\n4.   Wait Half Cycle\n5.   Set SCL = High\n6.   Wait Half Cycle\n7.   Set SDA = Low\n8.   Wait Half Cycle\n9.   Set SCL = Low\n10. Wait Half Cycle"
  # "Procedure: I2C-Send Stop Sequence\n1.   Set SCL = Low\n2.   Wait Half Cycle\n3.   Set SDA = Low\n4.   Wait Half Cycle\n5.   Set SCL = High\n6.   Wait Half Cycle\n7.   Set SDA = High\n8.   Wait Half Cycle\n9.   Set SCL = Low\n10. Wait Half Cycle"
  # "Procedure: I2C-Read Slave ACK\n1.  Set SCL = High (Start ACK Read)\n2.  Wait Half Cycle\n3.  Read SDA = Slave ACK\n4.  Wait Half Cycle\n5.  Set SCL = Low (End ACK Read)"
  # "Procedure: I2C-Receive Byte\n1.  Set Read Bits Remaining to 8\n2.  Set SCL = High (Start Bit Write)\n3.  Wait Half Cycle\n4.  Read SDA = Read Bit\n     Load Read Bit into Read FIFO\n     Decrement Read Bits Remaining\n5.  Wait Half Cycle\n6.  Set SCL = Low (End Bit Write)\n7.  Wait Half Cycle\n8.  If Read Bits Remaining = 0\n         Finished\n     If Read Bits Remaining > 0\n         Go to 2"
  # "Procedure: I2C-Send Data Byte\n1.  Set Write Bits Remaining = 8\n2.  Load Write Bit (U32) from Write FIFO\n3.  Set SDA = Write Bit (U32) [i] (i: 7 >> 0)\n     Decrement Write Bits Remaining\n4.  Wait Half Cycle\n5.  Set SCL = High (Start Bit Write)\n6.  Wait Half Cycle\n7.  Set Clock Low (End Bit Write)\n8.  Wait Half Cycle\n9.  If Write Bits Remaining = 0\n         Finished\n     If Write Bits Remaining > 0\n         Go to 2"
  # "Operation:  I2C-Read Data Bytes\nA:  Load Read Bytes Remaining with Bytes to Read\nB:  Procedure: I2C-Receive Byte\n      Decrement Read Bytes Remaining\n      If Read Bytes Remaining = 0\n          Set Master ACK = High\n      If Read Bytes Remaining > 0\n          Decrement Read Bytes Remaining\n          Set Master ACK = Low\nC:  Procedure: I2C-Write Master ACK\n      If Master ACK = High\n          Goto D\n      If Master ACK = Low\n          Go to B\nD:  Procedure: I2C-Send Stop Sequence"
  # "Operation:  I2C-Send Data Bytes\nA:  Read I2C Write FIFO\n      If Write FIFO Timed Out (No more Data)\n          Go to D\n      If Write FIFO Not Timed Out (Data Available)\n          Load Write Bits (U32)\n          Go to B\nB:  Procedure: I2C-Send Data Byte\nC:  Procedure: I2C-Read Slave ACK\n      Go to A\nD:   Procedure: I2C-Send Stop Sequence"
  # "Operation: I2C-Send Sub Address\nA:  Load Write Byte with Sub Address\nB:  Procedure: I2C-Send Address Byte\nC:  Procedure: I2C-Read Slave ACK"
  # "Procedures:\n\nI2C-Send Start Sequence\nI2C-Send Byte\nI2C-Read Slave ACK\nI2C-Write Master ACK\nI2C-Receive Byte\nI2C-Send Stop Sequence"
  # "Transaction: I2C-Write Data\n\nI.  Transfer Write Data Array to Write FIFO\nII.  Operation: I2C-Send Slave Address (W)\nIII.  Operation: I2C-Send Sub Address\nIV.  Operation: I2C-Send Data Bytes\nV.  Transfer Error Info to Status Array"
  # "Transaction: I2C-Read Data\n\nI.  Operation: I2C-Send Slave Address (W)\nII.  Operation: I2C-Send Sub Address\nIII.  Operation: I2C-Send Slave Address (R)\nIV.  Operation: I2C-Read Data Bytes\nV.  Transfer Read FIFO to Read Data Array\nVI.  Transfer Error Info to Status Array"
  # "Transactions:\n\nI2C-Read Data - Inputs[Slave Address, Sub Address, Bytes to Read]; Outputs[Read Data Array, Status Array]\nI2C-Write Data - Inputs[Slave Address, Sub Address, Write Data Array]; Outputs[Status Array]"
  # "Operations:\n\nI2C-Send Slave Address\nI2C-Send Sub Address\nI2C-Send Data Bytes\nI2C-Read Data Bytes"
  # "Operation: I2C-Send Slave Address\nA:  Procedure: I2C-Send Start Sequence\nB:  Load Write Byte [1-7] with Slave Address\nC:  Load Write Byte [0] with R/W Bit (0=Write, 1=Read)\nD:  Procedure: I2C-Send Addres Byte\nE:   Procedure: I2C-Read Slave ACK"
  n1 = flat-sequence {
    tunnel: [WSVCAP_SHL_Communication_Loop_State."Idle" ("Action")] -> w3
    tunnel: [w6] -> _
    frame #0 {
      w5 = WSVCAP_SHL_FIFO_Operation_Enum."Create FIFO/Memory" ("Operation")
      w7 = FALSE ("Done")
      # "Initialize"
      n2 = disable-structure shown="TARGET_TYPE==FPGA, Default" {
        disable-tunnel: [u32 1000 ("x-y") u32 40000000 ("x-y")] -> w6
        frame condition #0 {
          n3 = property on="Waveform Chart" class="WFChart (strict)"("History Data"=cluster{i16, i16, i16, i16}[] []) -> ()  [unwired: 2 in, 2 out]
        }
        frame condition #1 (active) {
        }
      }
      n4 = call "WSVCAP SHL FPGA LL I2C FIFO Manager - Pre and Post.vi"("Operation"=w5) -> ()  [unwired: 12 in, 3 out]
      n5 = call "FIFO Manager - Pre and Post.vi"("Operation"=w5) -> ()  [unwired: 12 in, 3 out]
      n6 = local write "Write Flag"(w7) -> ()
      n7 = local write "Read Flag"(w7) -> ()
      n8 = local write "Ack Read"(w7) -> ()
      n9 = local write "Start"(w7) -> ()
      n10 = local write "Exit"(w7) -> ()
      n11 = local write "Read Status Flag"(w7) -> ()
      n12 = local write "Ack Read Status"(w7) -> ()
      n13 = local write "Cmd"(WSVCAP_SHL_State."Idle" ("SPI_CMD_DBG")) -> ()
    }
  }
  n14 = while {
    shift-right: [w20] -> _
    shift-left: w3 -> [w27]
    shift-right: [w25] -> _
    shift-left: _ -> [w26]
    tunnel: [FALSE] -> w4
    shift-right: [w19] -> _
    shift-left: _ -> [w22]
    shift-left: w3 -> [w17]
    shift-right: [w16] -> _
    shift-left: 0 -> [w15]
    tunnel: u32 1000 ("x-y") -> [w14]
    i -> [w13]
    stop <- "Exit" stop-if-true
    # "Error Info"
    # "Main Loop"
    n15 = case shown="\"Transmit Data\"" w27 {
      tunnel: [w31 w46 WSVCAP_SHL_Communication_Loop_State."Transmit Data" ("Action") WSVCAP_SHL_Communication_Loop_State."Post Transmition" ("Action") WSVCAP_SHL_Communication_Loop_State."Operation Complete" ("Action") WSVCAP_SHL_Communication_Loop_State."Idle" ("Action")] -> w21
      tunnel: w26 -> [w28 w45 w79 w248 w617 w704]
      tunnel: [w28 w44 w78 w247 w616 w704] -> w25
      tunnel: [_ _ w81 w245 w624 _] -> w19
      tunnel: w22 -> [_ _ w86 w246 w625 w709]
      tunnel: w17 -> [_ _ _ _ _ w708]
      tunnel: [w29 w43 w82 w244 w621 _] -> w16
      tunnel: w15 -> [w29 w43 w83 _ w620 w706]
      tunnel: w14 -> [_ _ w85 _ w622 w705]
      tunnel: w13 -> [_ _ w84 _ _ _]
      frame "Idle" {
        # "Wait until Start Cmd is received from the host"
        n16 = case shown="True" "Start" {
          tunnel: [WSVCAP_SHL_Communication_Loop_State."Idle" ("Action") WSVCAP_SHL_Communication_Loop_State."Initialize" ("Action")] -> w31
          frame False {
            # "No Start Received - Keep waiting"
          }
          frame True {
            # "Start Received - Initiate Operation"
            n17 = local write "Start"(FALSE ("SPI_Start")) -> ()
          }
        }
      }
      frame "Initialize" {
        # "Load Values from Front Panel (Set by Host)"
        n18 = case shown="\"Transfer Data\"" "Cmd" {
          tunnel: [WSVCAP_SHL_Communication_Loop_State."Idle" ("Action") WSVCAP_SHL_Communication_Loop_State."Pre-Transmission" ("Action")] -> w46
          tunnel: w45 -> [w48 w69]
          tunnel: [w48 w70] -> w44
          tunnel: "Wait Ticks" -> [_ w57]
          tunnel: "Slave Address" -> [_ w55]
          tunnel: "Sub Address" -> [_ w68]
          tunnel: "Transaction" -> [_ w60]
          tunnel: "Bytes to Write" -> [_ w56]
          tunnel: "Bytes to Read" -> [_ w52]
          tunnel: "Socket Mask" -> [_ w67]
          tunnel: "UUT Set" -> [_ w53]
          frame "Idle" {
            # "This Case Should not Happen"
          }
          frame "Transfer Data" {
            w54 = FALSE ("Read Flag")
            w58 = TRUE ("Read Flag")
            # "Load Transfer State Machine Cluster"
            n19 = case shown="Default" w60 {
              tunnel: [WSVCAP_SHL_Transaction_Step_Enum."I2C Read - I:Send Slave Address (W)" ("Transaction Step") WSVCAP_SHL_Transaction_Step_Enum."I2C Write - I:Send Slave Address" ("Transaction Step") WSVCAP_SHL_Transaction_Step_Enum."SRL Write - I:Write Data" ("Transaction Step") WSVCAP_SHL_Transaction_Step_Enum."RFFE Ext Write - I.Write Data" ("Transaction Step")] -> w59
              frame "I2C-Read Data" {
              }
              frame "I2C-Write Data" {
              }
              frame "SRL-Write Data" {
              }
              frame Default {
              }
            }
            n20 = disable-structure shown="TARGET_TYPE!=FPGA" {
              frame condition #0 {
                n21 = global read "Debug Global.vi" "CH (1-24)"() -> (w76:i32)
                "Display CH (1-48)" <- w76
                n22 = global write "WSVCAP SHL FPGA LL RFFE Debug Global.vi" "RFFE CH (1-16)"(w76) -> ()
                n23 = global write "WSVCAP SHL FPGA LL I2C Debug Global.vi" "I2C CH (1-32)"(w76) -> ()
              }
              frame condition #1 (active) {
              }
            }
            n24 = local write "Read Flag"(w54) -> ()
            n25 = local write "Read Status Flag"(w54) -> ()
            n26 = Logical Shift(y=u8 3, x=w52) -> (x << y=w50:u8)
            n27 = Bundle By Name(cluster=w69, "UUT Set (0/1)"=w53, "Wait Ticks"=w57, "Read Bits Remaining"=w50, "Transaction"=w60, "Bytes to Write"=w56, "Bytes to Read"=w52, "Sub Address"=w68, "Socket Mask"=w67, "Transaction Step"=w59, "Slave Address"=w55, "Operation Step"=WSVCAP_SHL_Operation_Step_Enum."I2C Send Slave Add - A: Send Start Sequence", "Procedure Step"=WSVCAP_SHL_Procedure_Step_Enum."I2C Start/Stop - 1: Set Clock Low", "Write CMD Idx [0-95]"=u8 0 ("Write CMD [1-4]"), "Write Bit Index [0-18]"=u8 0 ("Write Bit Index [0-39]"), "Cycle Count"=u64 0 ("SPI Cycle Count"), "Wait Ticks Remaining"=u32 0, "Start Operation"=w58, "Start Procedure"=w58) -> (w70:T12)
          }
        }
      }
      frame "Pre-Transmission" {
        # "1 Second (ms)"
        # "Transfer All Data from Host into Write FIFO / Initialize Transfer State Machine and SRL Bus Data"
        n28 = disable-structure shown="TARGET_TYPE==FPGA, Default" {
          disable-tunnel: [_ i16 0] -> w77
          frame condition #0 {
            n29 = property on="Waveform Chart" class="WFChart (strict)"("History Data"=cluster{i16, i16, i16, i16}[] []) -> ()  [unwired: 2 in, 2 out]
          }
          frame condition #1 (active) {
          }
        }
        n30 = Unbundle By Name(w79) -> ("Bytes to Write"=w87:u8, "Transaction"=w80:T1)
        n31 = case shown="\"I2C-Write Data\", \"SRL-Write Data\"" w80 {
          selector: w80 -> [_ w103 _]
          tunnel: w87 -> [_ w98 _]
          tunnel: [w93 w109 w242] -> w81
          tunnel: w86 -> [w93 w108 w242]
          tunnel: w85 -> [_ w107 _]
          tunnel: w84 -> [_ w106 _]
          tunnel: w83 -> [w92 w105 _]
          tunnel: [w92 w104 _] -> w82
          tunnel: w79 -> [w91 w100 w243]
          tunnel: [w91 w99 w243] -> w78
          tunnel: w77 -> [_ _ _]
          frame "I2C-Read Data" {
            # "No Pre-Load Required for this operation"
          }
          frame "I2C-Write Data", "SRL-Write Data" {
            # "Bits"
            # "Bytes"
            # "Not I2C"
            # "SRL Cycle Already In Bits\nI2C Bytes to Bits"
            # "Load Write Data"
            n32 = To Long Integer(number=w98) -> (32bit integer=w96:i32)
            n33 = Greater Or Equal?(x=w103, y=WSVCAP_SHL_Transaction_Enum."RFFE-Ext Write" ("Transaction")) -> (x >= y?=w101:bool)
            n34 = Logical Shift(y=u8 3 ("x"), x=w96) -> (x << y=w95:i32)
            n35 = Select(t=w96, s=w101, f=w95) -> (s? t:f=w97:i32)
            n36 = for {
              N: w97 -> [w110]
              shift-right: [w127] -> w109
              shift-left: w108 -> [w125]
              tunnel: w103 -> [w123]
              tunnel: w107 -> [w121]
              tunnel: w106 -> [w120]
              shift-right: [w118] -> w104
              shift-left: w105 -> [w119]
              shift-right: [w112] -> w99
              shift-left: w100 -> [w113]
              i -> [w115]
              # "Fill up the FIFO/CMD and CMD Lengths with Write Data from the host"
              n37 = call "Tick Count"() -> ("Tick Count(mSec)"=w122:u32)
              n38 = flat-sequence {
                tunnel: [w135] -> w126
                tunnel: w125 -> [w136]
                tunnel: [w142] -> w124
                tunnel: w123 -> [w142]
                tunnel: w122 -> [w141]
                tunnel: w121 -> [w140]
                tunnel: w120 -> [w134]
                tunnel: w119 -> [w133]
                tunnel: [w132] -> w117
                tunnel: [w129] -> w116
                tunnel: w115 -> [w129]
                tunnel: [w131] -> w114
                tunnel: w113 -> [w131]
                tunnel: [w130] -> w111
                tunnel: w110 -> [w130]
                tunnel: [FALSE ("SPI_Write Flag")] -> w128
                tunnel: [w168] -> w127
                tunnel: w126 -> [w167]
                tunnel: w124 -> [w166]
                tunnel: [w165] -> w118
                tunnel: w117 -> [w165]
                tunnel: w116 -> [w164]
                tunnel: w114 -> [w163]
                tunnel: [w162] -> w112
                tunnel: w111 -> [w160]
                frame #0 {
                  # "Wait for Write Flag = True"
                  n39 = while {
                    tunnel: w141 -> [w157]
                    tunnel: w140 -> [w155]
                    tunnel: w136 -> [w154]
                    tunnel: ["Write Flag"] -> w139
                    tunnel: [w150] -> w138
                    stop <- w152 stop-if-true
                    n40 = Unbundle By Name(w154) -> ("status"=w153:bool)
                    n41 = call "Wait"("Count(mSec)"=u32 1 ("Count(Ticks)")) -> ("Tick Count(mSec)"=w158:u32)
                    n42 = Subtract(x=w158, y=w157) -> (x-y=w156:u32)
                    n43 = Greater?(x=w156, y=w155) -> (0:w150:bool)
                    n44 = Compound Arithmetic op=OR(w153, w150, "Write Flag") -> (w152:bool)
                  }
                  n45 = Compound Arithmetic op=AND(w138, invert w139) -> (w137:bool)
                  n46 = case shown="True" w137 {
                    selector: w137 -> [_ w148]
                    tunnel: [w144 w147] -> w135
                    tunnel: w136 -> [w144 w149]
                    tunnel: w134 -> [_ w145]
                    tunnel: [w143 w145] -> w132
                    tunnel: w133 -> [w143 _]
                    frame False {
                    }
                    frame True {
                      n47 = Bundle By Name(cluster=w149, "status"=w148, "code"=9901) -> (w147:errorcluster)
                    }
                  }
                }
                frame #1 {
                  # "Load Data from 'Write Data' Control"
                  n48 = case shown="\"SRL-Write Data\"" w166 {
                    tunnel: "Write Data" -> [w170 w175 w187]
                    tunnel: [w173 w178 w188] -> w168
                    tunnel: w167 -> [w172 w177 w189]
                    tunnel: w164 -> [_ _ w180]
                    tunnel: w163 -> [w171 w176 w185]
                    tunnel: [w171 w176 w186] -> w162
                    tunnel: w160 -> [_ _ w183]
                    frame "I2C-Write Data" {
                      # "Load Write Values into I2C Write FIFO"
                      n49 = call "WSVCAP SHL FPGA LL I2C FIFO Manager - Pre and Post.vi"("64 Bit Data In"=w170, "error in (no error)"=w172, "Operation"=WSVCAP_SHL_FIFO_Operation_Enum."Put Element in Write") -> ("error out"=w173:errorcluster)  [unwired: 10 in, 2 out]
                    }
                    frame Default {
                      # "Operations not Supported or No Pre-Load Required"
                      n50 = call "WSVCAP SHL FPGA LL I2C FIFO Manager - Pre and Post.vi"("64 Bit Data In"=w175, "error in (no error)"=w177, "Operation"=WSVCAP_SHL_FIFO_Operation_Enum."Put Element in Write") -> ("error out"=w178:errorcluster)  [unwired: 10 in, 2 out]
                    }
                    frame "SRL-Write Data" {
                      # "CMD Idx"
                      # "Iteration"
                      # "Load Registers"
                      n51 = Unbundle By Name(w185) -> ("Cycle Mode"=w184:bool)
                      n52 = Subtract(x=w180, y=1) -> (x-y=w181:i32)
                      n53 = case shown="1.." w180 {
                        selector: w180 -> [_ w210]
                        tunnel: w189 -> [w202 w215]
                        tunnel: [w202 w214] -> w188
                        tunnel: w187 -> [w204 w213]
                        tunnel: w185 -> [w201 w212]
                        tunnel: [w203 w211] -> w186
                        tunnel: w184 -> [_ w209]
                        tunnel: w183 -> [w197 _]
                        tunnel: w181 -> [_ w208]
                        frame ..0 {
                          # "No Read for SRL"
                          # "First Iteration - Set Cycle Mode, Load Number of Commands per Cycle"
                          n54 = To Unsigned Byte Integer(number=w197) -> (unsigned 8bit integer=w195:u8)
                          n55 = To Unsigned Long Integer(number=w204) -> (unsigned 32bit integer=w200:u32)
                          n56 = Subtract(x=w195, y=u8 9) -> (x-y=w192:u8)
                          n57 = Greater Than 0?(x=w200) -> (x > 0?=w199:bool)
                          n58 = Logical Shift(y=i8 -3, x=w192) -> (x << y=w191:u8)
                          n59 = Max & Min(x=w200, y=u32 1) -> (max(x,y)=w205:u32)  [unwired: 1 out]
                          n60 = Select(t=u8 0, s=w199, f=w191) -> (s? t:f=w194:u8)
                          n61 = To Unsigned Byte Integer(number=w205) -> (unsigned 8bit integer=w207:u8)
                          n62 = Bundle By Name(cluster=w201, "Read Bytes Remaining"=u8 0, "Bytes to Write"=w194, "Cycle Mode"=w199, "Commands per Cycle [1-96]"=w207) -> (w203:T12)
                        }
                        frame 1.. {
                          # "SRL Write - Load Commands and Delays into Storage"
                          n63 = case shown="True" w209 {
                            tunnel: w215 -> [w221 w230]
                            tunnel: [w220 w230] -> w214
                            tunnel: w213 -> [w216 w225]
                            tunnel: w212 -> [w217 w226]
                            tunnel: [w217 w232] -> w211
                            tunnel: w210 -> [_ w231]
                            tunnel: w208 -> [_ w224]
                            frame False {
                              # "Not Cycle Mode - Load FIFO"
                              n64 = To Unsigned Long Integer(number=w216) -> (unsigned 32bit integer=w218:u32)
                              n65 = call "FIFO Manager - Pre and Post.vi"("Word In"=w218, "error in (no error)"=w221, "Operation"=WSVCAP_SHL_FIFO_Operation_Enum."Put Element in Write") -> ("error out"=w220:errorcluster)  [unwired: 10 in, 2 out]
                            }
                            frame True {
                              # "Cycle Mode"
                              n66 = To Unsigned Long Integer(number=w224) -> (unsigned 32bit integer=w223:u32)
                              n67 = Split Number(x=w225) -> (hi(x)=w227:u32, lo(x)=w228:u32)
                              n68 = call "Manage Cycle Memory.vi"("Operation"=MISC_IO_Choice_Enum."Write", "Address"=w223, "Write Data"=w225) -> ()  [unwired: 8 in, 1 out]
                              n69 = To Unsigned Quad Integer(1:w228) -> (0:w229:u64)
                              n70 = case shown="1" w231 {
                                tunnel: [w233 w240] -> w232
                                tunnel: w226 -> [w233 w241]
                                tunnel: w229 -> [_ w239]
                                tunnel: w227 -> [_ w235]
                                frame Default {
                                # "Load Idx 1.. into Buffer"
                                }
                                frame 1 {
                                # "Load First CMD"
                                n71 = Bundle By Name(cluster=w241, "CMD Length [1-48]"=u8 19, "CMD Delay (Ticks)"=w235, "Cycle CMD"=w239, "Write CMD Idx [0-95]"=u8 0 ("Write CMD [1-4]"), "Cycle Count"=u64 0, "Write Bit Index [0-18]"=u8 0) -> (w240:T12)
                                }
                              }
                            }
                          }
                        }
                      }
                    }
                  }
                }
              }
              n72 = local write "Write Flag"(w128) -> ()
            }
          }
          frame Default {
            # "Operations not Supported or No Pre-Load Required"
          }
        }
      }
      frame "Transmit Data" {
        # "Perform Write/Read Operation for All Bytes"
        n73 = node-c288() -> (w250:T9)  [unwired: 1 out]
        n74 = timed-loop {
          timing-out: [_] -> w249
          timing: w250 -> [_]
          shift-right: [w277] -> w247
          shift-left: w248 -> [w285]
          tunnel: w246 -> [w282]
          tunnel: [w279] -> w245
          tunnel: [w289] -> w244
          stop <- w290 stop-if-true
          # "Stop Cycle"
          # "Cmd per Cycle"
          # "Write CMD (1-4)"
          # "LD CMD"
          # "Transaction"
          # "Transaction"
          # "Transaction Finished"
          # "Procedure Finished"
          # "Next Operation Step"
          # "Operation Finished"
          # "Procedure Finished"
          # "Operation Finished"
          # "Next Operation Step"
          # "Procedure Finished"
          # "Operation Step"
          # "Cycle Mode"
          # "CMD Delay (Ticks)"
          # "Transaction Step"
          # "Send Digital Data (CLK | DAT | SYNC | EN | Etc.)"
          n75 = call "WSVCAP SHL FPGA LL Manage Initial States.vi"("Transfer Cluster In"=w285) -> ("Transfer Cluster Out"=w283:T12)  [unwired: 14 in]
          n76 = Unbundle By Name(w283) -> ("Transaction"=w287:T1, "Transaction Step"=w286:T7, "Procedure"=w284:T13, "Bytes to Read"=w254:u8, "CMD Length [1-48]"=w262:u8, "CMD Delay (Ticks)"=w261:u32, "Start Procedure"=w272:bool, "Wait Ticks Remaining"=w271:u32, "Procedure Step"=w270:T5, "Wait Ticks"=w269:u32, "Write Bits Remaining"=w268:u8, "Write Byte"=w267:u8, "Read Bits Remaining"=w265:u8, "Read Bytes Remaining"=w253:u8, "Write Bit Index [0-18]"=w263:u8, "Cycle Mode"=w260:bool, "Cycle CMD"=w264:u64, "Socket Mask"=w266:u32, "Operation Step"=w255:T6, "Write CMD Idx [0-95]"=w256:u8, "Commands per Cycle [1-96]"=w257:u8, "UUT Set (0/1)"=w252:u8)
          n77 = case "Execute Procedure" shown="\"SRL-Wait CMD Delay\"" w284 {
            tunnel: w282 -> [w438 w454 w469 w483 w495 w511 w525 w533 w551 w570 w575]
            tunnel: [w438 w453 w468 w482 w494 w510 w524 w532 w550 w569 w575] -> w281
            tunnel: [TRUE ("Finished") w452 w462 w481 w493 w505 w523 TRUE ("Finished") w535 w556 TRUE ("Finished")] -> w274
            tunnel: w283 -> [w439 w449 w467 w480 w491 w509 w517 w531 w549 w564 w576]
            tunnel: [w439 w450 w466 w479 w492 w508 w516 w530 w548 w563 w576] -> w259
            tunnel: w261 -> [_ _ _ _ _ _ _ _ _ w565 _]
            tunnel: w272 -> [_ _ _ _ _ _ _ _ _ w557 _]
            tunnel: w271 -> [_ w445 w464 w475 w486 w507 w520 _ w545 w567 _]
            tunnel: w270 -> [_ w447 w460 w474 w489 w501 w519 _ w546 _ _]
            tunnel: w269 -> [_ w443 w459 w473 w488 w500 w518 _ w540 _ _]
            tunnel: w266 -> [_ w442 w456 w471 w487 w497 w521 w526 w538 w553 _]
            tunnel: w268 -> [_ _ w458 w472 _ _ _ _ _ _ _]
            tunnel: w267 -> [_ _ w457 _ _ _ _ _ _ _ _]
            tunnel: w265 -> [_ _ _ _ _ w499 _ _ _ _ _]
            tunnel: w253 -> [_ _ _ _ _ w498 w513 _ _ _ _]
            tunnel: w264 -> [_ _ _ _ _ _ _ _ w547 _ _]
            tunnel: w260 -> [_ _ _ _ _ _ _ w529 w536 _ _]
            tunnel: w263 -> [_ _ _ _ _ _ _ _ w539 _ _]
            tunnel: w262 -> [_ _ _ _ _ _ _ _ w544 _ _]
            tunnel: "Stop Cycle" -> [_ _ _ _ _ _ _ w528 _ w554 _]
            tunnel: w257 -> [_ _ _ _ _ _ _ _ _ w561 _]
            tunnel: w256 -> [_ _ _ _ _ _ _ _ _ w559 _]
            tunnel: w255 -> [_ w441 _ _ _ _ _ _ _ _ _]
            tunnel: w254 -> [_ _ _ _ _ _ _ _ _ _ _]
            tunnel: w252 -> [_ w440 w455 w470 w484 w496 w512 _ _ _ _]
            frame "None" {
            }
            frame "I2C-Send Start/Stop Sequence" {
              n78 = Equal?(x=w441, y=WSVCAP_SHL_Operation_Step_Enum."I2C Send Slave Add - A: Send Start Sequence" ("Operation Step")) -> (x = y?=w448:bool)
              n79 = call "WSVCAP SHL FPGA LL Procedure I2C - Send Start or Stop Sequence.vi"("Procedure Step"=w447, "Wait Ticks Remaining"=w445, "I2C Wait Ticks"=w443, "error in (no error)"=w454, "Type (T:Start; F:Stop)"=w448, "Socket Mask"=w442, "UUT Set (0/1)"=w440) -> ("Wait Ticks Remaining Out"=w444:u32, "Procedure Step Out"=w446:T5, "Finished"=w452:bool, "error out"=w453:errorcluster)  [unwired: 5 in]
              n80 = Bundle By Name(cluster=w449, "Wait Ticks Remaining"=w444, "Procedure Step"=w446) -> (w450:T12)
            }
            frame "I2C-Send Address Byte" {
              n81 = call "WSVCAP SHL FPGA LL Procedure I2C - Send Address Byte.vi"("Procedure Step"=w460, "Wait Ticks Remaining"=w464, "I2C Wait Ticks"=w459, "Write Bits Remaining"=w458, "Write Byte"=w457, "error in (no error)"=w469, "Socket Mask"=w456, "UUT Set (0/1)"=w455) -> ("Wait Ticks Remaining Out"=w463:u32, "Procedure Step Out"=w465:T5, "Write Bits Remaining Out"=w461:u8, "Finished"=w462:bool, "error out"=w468:errorcluster)  [unwired: 3 in]
              n82 = Bundle By Name(cluster=w467, "Wait Ticks Remaining"=w463, "Procedure Step"=w465, "Write Bits Remaining"=w461) -> (w466:T12)
            }
            frame "I2C-Send Data Byte" {
              n83 = call "WSVCAP SHL FPGA LL I2C Procedure - Send Data Byte.vi"("Procedure Step"=w474, "Wait Ticks Remaining"=w475, "I2C Wait Ticks"=w473, "Write Bits Remaining"=w472, "error in (no error)"=w483, "Socket Mask"=w471, "UUT (0/1)"=w470) -> ("Wait Ticks Remaining Out"=w478:u32, "Procedure Step Out"=w477:T5, "Write Bits Remaining Out"=w476:u8, "Finished"=w481:bool, "error out"=w482:errorcluster)  [unwired: 4 in]
              n84 = Bundle By Name(cluster=w480, "Wait Ticks Remaining"=w478, "Procedure Step"=w477, "Write Bits Remaining"=w476) -> (w479:T12)
            }
            frame "I2C-Read ACK" {
              n85 = call "WSVCAP SHL FPGA LL Procedure I2C - Read ACK.vi"("Procedure Step"=w489, "Wait Ticks Remaining"=w486, "I2C Wait Ticks"=w488, "Socket Mask"=w487, "error in (no error)"=w495, "UUT Set (0/1)"=w484) -> ("Wait Ticks Remaining Out"=w485:u32, "Procedure Step Out"=w490:T5, "Finished"=w493:bool, "error out"=w494:errorcluster)  [unwired: 5 in, 1 out]
              n86 = Bundle By Name(cluster=w491, "Wait Ticks Remaining"=w485, "Procedure Step"=w490) -> (w492:T12)
            }
            frame "I2C-Receive Byte" {
              n87 = call "WSVCAP SHL FPGA LL Procedure I2C - Receive Byte.vi"("Procedure Step"=w501, "Wait Ticks Remaining"=w507, "I2C Wait Ticks"=w500, "Read Bits Remaining"=w499, "Read Bytes Remaining"=w498, "error in (no error)"=w511, "Socket Mask"=w497, "UUT Set (0/1)"=w496) -> ("Wait Ticks Remaining Out"=w506:u32, "Procedure Step Out"=w504:T5, "Finished"=w505:bool, "Read Bits Remaining Out"=w503:u8, "Read Bytes Remaining Out"=w502:u8, "error out"=w510:errorcluster)  [unwired: 2 in]
              n88 = Bundle By Name(cluster=w509, "Wait Ticks Remaining"=w506, "Procedure Step"=w504, "Read Bits Remaining"=w503, "Read Bytes Remaining"=w502) -> (w508:T12)
            }
            frame "I2C-Write ACK" {
              n89 = Less Or Equal To 0?(x=w513) -> (x <= 0?=w522:bool)
              n90 = call "WSVCAP SHL FPGA LL Procedure I2C - Send ACK.vi"("Procedure Step"=w519, "Wait Ticks Remaining"=w520, "I2C Wait Ticks"=w518, "ACK Bit to Write"=w522, "error in (no error)"=w525, "Socket Mask"=w521, "UUT (0/1)"=w512) -> ("Wait Ticks Remaining Out"=w515:u32, "Procedure Step Out"=w514:T5, "Finished"=w523:bool, "error out"=w524:errorcluster)  [unwired: 5 in]
              n91 = Bundle By Name(cluster=w517, "Wait Ticks Remaining"=w515, "Procedure Step"=w514) -> (w516:T12)
            }
            frame "SRL-Clear Lines" {
              n92 = Compound Arithmetic op=AND(w529, invert w528) -> (w527:bool)
              n93 = Bundle By Name(cluster=w531, "Cycle Mode"=w527) -> (w530:T12)
              n94 = call "Procedure - Clear Lines.vi"("error in (no error)"=w533, "Socket Mask"=w526) -> ("error out"=w532:errorcluster)  [unwired: 13 in]
            }
            frame "SRL-Send Data" {
              n95 = call "Procedure - Send Data.vi"("Procedure Step"=w546, "Wait Ticks Remaining"=w545, "CMD Length [1-40]"=w544, "SRL Wait Ticks"=w540, "Write Bit Index [0-18]"=w539, "SRL Cycle Mode"=w536, "error in (no error)"=w551, "SRL Cycle CMD"=w547, "Socket Mask"=w538) -> ("Wait Ticks Remaining Out"=w543:u32, "Procedure Step Out"=w542:T5, "Write Bit Index [0-18] Out"=w541:u8, "Finished"=w535:bool, "error out"=w550:errorcluster)  [unwired: 2 in]
              n96 = Bundle By Name(cluster=w549, "Wait Ticks Remaining"=w543, "Procedure Step"=w542, "Write Bit Index [0-18]"=w541, "CMD Length [1-48]"=u8 19) -> (w548:T12)
            }
            frame "SRL-Wait CMD Delay" {
              # "Last Tick"
              # "First Tick"
              n97 = Decrement(x=w561) -> (x-1=w552:u8)
              n98 = Select(t=w565, s=w557, f=w567) -> (s? t:f=w566:u32)
              n99 = Equal?(x=w559, y=w552) -> (x = y?=w560:bool)
              n100 = Decrement(x=w566) -> (x-1=w568:u32)
              n101 = Compound Arithmetic op=AND(w560, w554) -> (w558:bool)
              n102 = Less Or Equal To 0?(x=w568) -> (x <= 0?=w556:bool)
              n103 = Compound Arithmetic op=AND(w556, invert w558) -> (w555:bool)
              n104 = Bundle By Name(cluster=w564, "Wait Ticks Remaining"=w568) -> (w563:T12)
              n105 = Compound Arithmetic op=OR(w555, w557) -> (w562:bool)
              n106 = case shown="True" w562 {
                tunnel: w570 -> [w571 w574]
                tunnel: [w571 w573] -> w569
                tunnel: w553 -> [_ w572]
                frame False {
                }
                frame True {
                  # "First or Last Tick of Wait Cycle"
                  n107 = call "Procedure - Clear Lines.vi"("error in (no error)"=w574, "Socket Mask"=w572) -> ("error out"=w573:errorcluster)  [unwired: 13 in]
                }
              }
            }
            frame Default {
            }
          }
          n108 = case "Post-Procedure" shown="\"SRL Write Data - B: Wait CMD Delay\"" w255 {
            selector: w255 -> [w330 w333 w338 w339 w343 w347 w350 _ w357 w370 w371 w375 w377 w387 w391 w410 w428 w431 w435]
            tunnel: [w328 w332 w336 w340 w344 w349 w352 w354 w359 w366 w373 w376 w381 w390 w393 w414 w429 w432 w436] -> w279
            tunnel: w281 -> [w328 w332 w336 w340 w344 w349 w352 w354 w359 w367 w373 w376 w381 w390 w393 w414 w429 w432 w436]
            tunnel: [_ _ _ w341 _ _ w351 _ _ _ w372 _ _ _ w392 _ _ w430 TRUE ("Finished")] -> w273
            tunnel: w274 -> [w327 _ w335 w341 _ w346 w351 _ w355 w368 w372 _ w379 w389 w392 w396 w416 w430 _]
            tunnel: [w326 w331 w334 w339 w342 w345 w350 WSVCAP_SHL_Operation_Step_Enum."I2C Send Data - B: Send Data Byte" ("Operation Step") w356 w369 w371 w374 w378 w388 w391 w413 w427 w431 w433] -> w275
            tunnel: [_ _ _ _ _ _ _ _ _ _ _ _ _ _ _ w398 w418 _ _] -> w280
            tunnel: w261 -> [_ _ _ _ _ _ _ _ _ _ _ _ _ _ _ w404 _ _ _]
            tunnel: w260 -> [_ _ _ _ _ _ _ _ _ _ _ _ _ _ _ w397 w417 _ _]
            tunnel: "Stop Cycle" -> [_ _ _ _ _ _ _ _ _ _ _ _ _ _ _ w399 w421 _ _]
            tunnel: w256 -> [_ _ _ _ _ _ _ _ _ _ _ _ _ _ _ w403 w423 _ _]
            tunnel: w257 -> [_ _ _ _ _ _ _ _ _ _ _ _ _ _ _ w402 w422 _ _]
            tunnel: w253 -> [_ _ _ _ _ _ _ _ _ _ _ _ _ w382 _ _ _ _ _]
            frame "I2C Send Slave Add - A: Send Start Sequence" {
              n109 = Increment(x=w330) -> (x+1=w329:T6)
              n110 = Select(t=w329, s=w327, f=w330) -> (s? t:f=w326:T6)
            }
            frame "I2C Send Slave Add - B: Load Address Byte" {
              n111 = Increment(x=w333) -> (x+1=w331:T6)
            }
            frame "I2C Send Slave Add - C: Send Address Byte" {
              n112 = Increment(x=w338) -> (x+1=w337:T6)
              n113 = Select(t=w337, s=w335, f=w338) -> (s? t:f=w334:T6)
            }
            frame "I2C Send Slave Add - D: Read Slave ACK" {
            }
            frame "I2C Send Sub Add - A: Load Sub Address" {
              n114 = Increment(x=w343) -> (x+1=w342:T6)
            }
            frame "I2C Send Sub Add - B: Send Address Byte" {
              n115 = Increment(x=w347) -> (x+1=w348:T6)
              n116 = Select(t=w348, s=w346, f=w347) -> (s? t:f=w345:T6)
            }
            frame "I2C Send Sub Add - C: Read Slave ACK" {
            }
            frame "I2C Send Data - A: Get Byte from FIFO" {
            }
            frame "I2C Send Data - B: Send Data Byte" {
              n117 = Increment(x=w357) -> (x+1=w358:T6)
              n118 = Select(t=w358, s=w355, f=w357) -> (s? t:f=w356:T6)
            }
            frame "I2C Send Data - C: Read Slave ACK" {
              n119 = call "WSVCAP SHL FPGA LL I2C FIFO Manager - Transfer.vi"("error in (no error)"=w367, "Operation"=WSVCAP_SHL_FIFO_Operation_Enum."Get Write FIFO Status") -> ("Data Out"=w364:u64, "error out"=w366:errorcluster)  [unwired: 11 in, 1 out]
              n120 = Equal To 0?(x=w364) -> (x = 0?=w363:bool)
              n121 = Select(t=WSVCAP_SHL_Operation_Step_Enum."I2C Send Data - D: Send Stop Sequence" ("Operation Step"), s=w363, f=WSVCAP_SHL_Operation_Step_Enum."I2C Send Data - A: Get Byte from FIFO" ("Operation Step")) -> (s? t:f=w360:T6)
              n122 = Select(t=w360, s=w368, f=w370) -> (s? t:f=w369:T6)
            }
            frame "I2C Send Data - D: Send Stop Sequence" {
            }
            frame "I2C Read Data - A: Load Bytes to Read" {
              n123 = Increment(x=w375) -> (x+1=w374:T6)
            }
            frame "I2C Read Data - B: Receive Byte" {
              n124 = Increment(x=w377) -> (x+1=w380:T6)
              n125 = Select(t=w380, s=w379, f=w377) -> (s? t:f=w378:T6)
            }
            frame "I2C Read Data - C: Write Master ACK" {
              n126 = Less Or Equal To 0?(x=w382) -> (x <= 0?=w383:bool)
              n127 = Increment(x=w387) -> (x+1=w385:T6)
              n128 = Select(t=w385, s=w383, f=WSVCAP_SHL_Operation_Step_Enum."I2C Read Data - B: Receive Byte" ("Operation Step")) -> (s? t:f=w384:T6)
              n129 = Select(t=w384, s=w389, f=w387) -> (s? t:f=w388:T6)
            }
            frame "I2C Read Data - D: Send Stop Sequence" {
            }
            frame "SRL Write Data - A: Send Data" {
              n130 = Equal To 0?(x=w404) -> (x = 0?=w395:bool)
              n131 = Decrement(x=w402) -> (x-1=w394:u8)
              n132 = Equal?(x=w403, y=w394) -> (x = y?=w401:bool)
              n133 = Compound Arithmetic op=AND(w401, w399) -> (w400:bool)
              n134 = Compound Arithmetic op=AND(w397, w395, w396) -> (w398:bool)
              n135 = Select(t=WSVCAP_SHL_Operation_Step_Enum."SRL Write Data - A: Send Data" ("Operation Step"), s=w395, f=WSVCAP_SHL_Operation_Step_Enum."SRL Write Data - B: Wait CMD Delay" ("Operation Step")) -> (s? t:f=w407:T6)
              n136 = Select(t=WSVCAP_SHL_Operation_Step_Enum."SRL Write Data - C: Clear Lines" ("Operation Step"), s=w400, f=w407) -> (s? t:f=w406:T6)
              n137 = Select(t=w406, s=w397, f=WSVCAP_SHL_Operation_Step_Enum."SRL Write Data - C: Clear Lines" ("Operation Step")) -> (s? t:f=w412:T6)
              n138 = Select(t=w412, s=w396, f=w410) -> (s? t:f=w413:T6)
            }
            frame "SRL Write Data - B: Wait CMD Delay" {
              n139 = Decrement(x=w422) -> (x-1=w415:u8)
              n140 = Equal?(x=w423, y=w415) -> (x = y?=w420:bool)
              n141 = Compound Arithmetic op=AND(w420, w421) -> (w419:bool)
              n142 = Select(t=WSVCAP_SHL_Operation_Step_Enum."SRL Write Data - C: Clear Lines" ("f"), s=w419, f=WSVCAP_SHL_Operation_Step_Enum."SRL Write Data - A: Send Data") -> (s? t:f=w425:T6)
              n143 = Compound Arithmetic op=AND(w416, w417) -> (w418:bool)
              n144 = Select(t=w425, s=w416, f=w428) -> (s? t:f=w427:T6)
            }
            frame "SRL Write Data - C: Clear Lines" {
            }
            frame Default {
              n145 = Increment(x=w435) -> (x+1=w433:T6)
            }
          }
          n146 = case shown="True" w280 {
            tunnel: w259 -> [w322 w325]
            tunnel: [w322 w324] -> w278
            frame False {
            }
            frame True {
              # "Load next SRL\nCycle CMD"
              n147 = call "Load Next Cycle CMD.vi"("Transfer Cluster In"=w325) -> ("Transfer Cluster Out"=w324:T12, "SRL Cycle Count"=→"Cycle Count":u64)  [unwired: 13 in]
            }
          }
          n148 = case "Post Operation" shown="\"SRL Write - I:Write Data\"" w286 {
            selector: w286 -> [w294 w298 w301 w304 w308 w312 w317 w319 w321]
            tunnel: [_ _ w300 _ _ _ w316 w318 TRUE ("Finished")] -> w288
            tunnel: w273 -> [w292 w296 w300 w303 w307 w311 w316 w318 _]
            tunnel: [w295 w299 w301 w302 w306 w310 w314 w319 w321] -> w276
            frame "I2C Write - I:Send Slave Address" {
              n149 = Increment(x=w294) -> (x+1=w293:T7)
              n150 = Select(t=w293, s=w292, f=w294) -> (s? t:f=w295:T7)
            }
            frame "I2C Write - II:Send Sub Address" {
              n151 = Increment(x=w298) -> (x+1=w297:T7)
              n152 = Select(t=w297, s=w296, f=w298) -> (s? t:f=w299:T7)
            }
            frame "I2C Write - III:Send Data Bytes" {
            }
            frame "I2C Read - I:Send Slave Address (W)" {
              n153 = Increment(x=w304) -> (x+1=w305:T7)
              n154 = Select(t=w305, s=w303, f=w304) -> (s? t:f=w302:T7)
            }
            frame "I2C Read - II:Send Sub Address" {
              n155 = Increment(x=w308) -> (x+1=w309:T7)
              n156 = Select(t=w309, s=w307, f=w308) -> (s? t:f=w306:T7)
            }
            frame "I2C Read - III:Send Slave Address (R)" {
              n157 = Increment(x=w312) -> (x+1=w313:T7)
              n158 = Select(t=w313, s=w311, f=w312) -> (s? t:f=w310:T7)
            }
            frame "I2C Read - IV:Read Data Bytes" {
              n159 = Select(t=WSVCAP_SHL_Transaction_Step_Enum."I2C Read - I:Send Slave Address (W)" ("Transaction Step"), s=w316, f=w317) -> (s? t:f=w314:T7)
            }
            frame "SRL Write - I:Write Data" {
            }
            frame Default {
            }
          }
          n160 = Bundle By Name(cluster=w278, "Transaction Step"=w276, "Operation Step"=w275, "Start Operation"=w273, "Start Procedure"=w274) -> (w277:T12)
          n161 = disable-structure shown="TARGET_TYPE!=FPGA, Default" {
            disable-tunnel: w287 -> [w578 _]
            disable-tunnel: w288 -> [_ _]
            frame condition #0 {
              n162 = case shown="Default" w578 {
                tunnel: [w585 w594 w604] -> w579
                frame "RFFE-Ext Write", "RFFE-Ext Read" {
                  n163 = global read "WSVCAP SHL FPGA LL RFFE Debug Global.vi" "RFFE_CLK"() -> (w584:bool)
                  n164 = global read "WSVCAP SHL FPGA LL RFFE Debug Global.vi" "RFFE_DAA"() -> (w583:bool)
                  n165 = global read "WSVCAP SHL FPGA LL RFFE Debug Global.vi" "RFFE_CLK"() -> (w588:bool)
                  n166 = global read "WSVCAP SHL FPGA LL RFFE Debug Global.vi" "RFFE_DATO"() -> (w581:bool)
                  n167 = Boolean To (0,1)(Boolean=w584) -> (0, 1=w590:i16)
                  n168 = Boolean To (0,1)(Boolean=w583) -> (0, 1=w589:i16)
                  n169 = Boolean To (0,1)(Boolean=w588) -> (0, 1=w582:i16)
                  n170 = Boolean To (0,1)(Boolean=w581) -> (0, 1=w580:i16)
                  n171 = Bundle(w590, w589, w582, w580) -> (w587:cluster{i16, i16, i16, i16})  [unwired: 1 in]
                  n172 = Add(x=w587, y=cluster{i16, i16, i16, i16} {0, 2, 4, 6} ("Waveform Chart")) -> (x+y=w585:cluster{i16, i16, i16, i16})
                }
                frame Default {
                  w593 = i16 0 ("0, 1")
                  n173 = global read "WSVCAP SHL FPGA LL I2C Debug Global.vi" "I2C SCL"() -> (w592:bool)
                  n174 = global read "WSVCAP SHL FPGA LL I2C Debug Global.vi" "I2C SDA"() -> (w591:bool)
                  n175 = Boolean To (0,1)(Boolean=w592) -> (0, 1=w598:i16)
                  n176 = Boolean To (0,1)(Boolean=w591) -> (0, 1=w597:i16)
                  n177 = Bundle(w598, w597, "0, 1"=w593, "0, 1"=w593) -> (w596:cluster{i16, i16, "0, 1":i16, "0, 1":i16})  [unwired: 1 in]
                  n178 = Add(x=w596, y=cluster{i16, i16, i16, i16} {0, 2, -1, -1} ("Waveform Chart")) -> (x+y=w594:cluster{i16, i16, i16, i16})
                }
                frame "SRL-Write Data" {
                  n179 = global read "Debug Global.vi" "DIN"() -> (w601:bool)
                  n180 = global read "Debug Global.vi" "SCLK"() -> (w602:bool)
                  n181 = global read "Debug Global.vi" "SYNC"() -> (w600:bool)
                  n182 = Boolean To (0,1)(Boolean=w602) -> (0, 1=w608:i16)
                  n183 = Boolean To (0,1)(Boolean=w601) -> (0, 1=w607:i16)
                  n184 = Boolean To (0,1)(Boolean=w600) -> (0, 1=w599:i16)
                  n185 = Bundle(w608, w607, w599, "0, 1"=i16 0) -> (w606:cluster{i16, i16, i16, "0, 1":i16})  [unwired: 1 in]
                  n186 = Add(x=w606, y=cluster{i16, i16, i16, i16} {0, 2, 4, -1} ("Waveform Chart")) -> (x+y=w604:cluster{i16, i16, i16, i16})
                }
              }
              "Waveform Chart" <- w579
            }
            frame condition #1 (active) {
            }
          }
          n187 = Unbundle By Name(w279) -> ("status"=w291:bool)
          n188 = To Long Integer(number=w287) -> (32bit integer=w289:i32)
          n189 = Compound Arithmetic op=OR(w288, w291) -> (w290:bool)
        }
        n190 = node-c288(w249) -> ()
      }
      frame "Post Transmition" {
        # "1 Second (Ticks)"
        # "Error Info"
        # "Transfer Data from Read FIFO to Host"
        n191 = Unbundle By Name(w617) -> ("Cycle Count"=w614:u64, "Cycle Mode"=w615:bool, "Bytes to Read"=w619:u8, "Transaction"=w623:T1)
        n192 = Increment(x=w614) -> (x+1=w618:u64)
        n193 = Select(t=w618, s=w615, f=w614) -> (s? t:f=w613:u64)
        n194 = Bundle By Name(cluster=w617, "Cycle Count"=w613) -> (w616:T12)
        n195 = case shown="1.." w619 {
          selector: w619 -> [_ w632]
          tunnel: w625 -> [w628 w638]
          tunnel: [w628 w637] -> w624
          tunnel: w623 -> [_ w636]
          tunnel: w622 -> [_ w635]
          tunnel: [w627 w634] -> w621
          tunnel: w620 -> [w627 w633]
          frame ..0 {
            # "No Read Operation"
          }
          frame 1.. {
            # "Transfer Read Data"
            # "Read all data and transfer to the host"
            n196 = Logical Shift(y=u8 3, x=w632) -> (x << y=w630:u8)
            n197 = To Long Integer(number=w630) -> (32bit integer=w629:i32)
            n198 = for {
              N: w629 -> [_]
              shift-right: [w654] -> w637
              shift-left: w638 -> [w655]
              tunnel: w636 -> [w651]
              tunnel: w635 -> [w650]
              shift-right: [w641] -> w634
              shift-left: w633 -> [w639]
              i -> [w644]
              n199 = flat-sequence {
                tunnel: w655 -> [w662]
                tunnel: [w661] -> w652
                tunnel: w651 -> [w659]
                tunnel: w650 -> [w658]
                tunnel: [w658] -> w649
                tunnel: [w657] -> w645
                tunnel: w644 -> [w657]
                tunnel: [w656] -> w642
                tunnel: w639 -> [w656]
                tunnel: [w671] -> w653
                tunnel: w652 -> [w671]
                tunnel: w649 -> [w670]
                tunnel: [w670] -> w648
                tunnel: [w669] -> w646
                tunnel: w645 -> [w669]
                tunnel: [w668] -> w643
                tunnel: w642 -> [w668]
                tunnel: w653 -> [w680]
                tunnel: w648 -> [w681]
                tunnel: [w679] -> w647
                tunnel: w646 -> [w675]
                tunnel: w643 -> [w674]
                tunnel: [w673] -> w640
                tunnel: [w701] -> w654
                tunnel: w647 -> [w701]
                tunnel: [w700] -> w641
                tunnel: w640 -> [w700]
                frame #0 {
                  n200 = case shown="\"RFFE-Ext Write\".." w659 {
                    tunnel: w662 -> [w666 w667]
                    tunnel: [w665 w667] -> w661
                    tunnel: [w664 _] -> w660
                    frame "I2C-Read Data", "I2C-Write Data" {
                      n201 = call "WSVCAP SHL FPGA LL I2C FIFO Manager - Pre and Post.vi"("error in (no error)"=w666, "Operation"=WSVCAP_SHL_FIFO_Operation_Enum."Get Element from Read") -> ("64 Bit Data Out"=w664:u64, "error out"=w665:errorcluster)  [unwired: 11 in, 1 out]
                    }
                    frame "RFFE-Ext Write".. {
                    }
                  }
                  "Read Data" <- w660
                }
                frame #1 {
                  "Read Flag" <- TRUE ("Read Flag")
                }
                frame #2 {
                  n202 = call "Tick Count2"() -> ("Tick Count(mSec)"=w682:u32)
                  n203 = while {
                    tunnel: w682 -> [w697]
                    tunnel: w681 -> [w695]
                    tunnel: w680 -> [w694]
                    tunnel: ["Ack Read"] -> w677
                    tunnel: [w691] -> w678
                    stop <- w692 stop-if-true
                    n204 = Unbundle By Name(w694) -> ("status"=w693:bool)
                    n205 = call "Wait2"("Count(mSec)"=u32 1 ("Count(Ticks)")) -> ("Tick Count(mSec)"=w698:u32)
                    n206 = Subtract(x=w698, y=w697) -> (x-y=w696:u32)
                    n207 = Greater?(x=w696, y=w695) -> (0:w691:bool)
                    n208 = Compound Arithmetic op=OR(w693, w691, "Ack Read") -> (w692:bool)
                  }
                  n209 = Compound Arithmetic op=AND(w678, invert w677) -> (w676:bool)
                  n210 = case shown="True" w676 {
                    selector: w676 -> [_ w688]
                    tunnel: [w684 w687] -> w679
                    tunnel: w680 -> [w684 w689]
                    tunnel: [w683 w685] -> w673
                    tunnel: w675 -> [_ w685]
                    tunnel: w674 -> [w683 _]
                    frame False {
                    }
                    frame True {
                      n211 = Bundle By Name(cluster=w689, "status"=w688, "code"=9902) -> (w687:errorcluster)
                    }
                  }
                }
                frame #3 {
                  n212 = local write "Ack Read"(FALSE ("Read Flag")) -> ()
                }
              }
            }
          }
        }
      }
      frame "Operation Complete" {
        # "Transfer Status"
        n213 = Unbundle By Name(w704) -> ("Cycle Mode"=w703:bool)
        n214 = To Long Integer(number=w708) -> (32bit integer=w707:i32)
        n215 = case shown="False" w703 {
          tunnel: w709 -> [w716 _]
          tunnel: w707 -> [w715 _]
          tunnel: w706 -> [w714 _]
          tunnel: w705 -> [w712 _]
          frame False {
            # "Return Status"
            n216 = for {
              N: 4 -> [_]
              tunnel: w716 -> [w723]
              tunnel: w715 -> [w722]
              tunnel: w714 -> [w721]
              tunnel: w712 -> [w717]
              i -> [w720]
              n217 = flat-sequence {
                tunnel: w723 -> [w733]
                tunnel: w722 -> [w726]
                tunnel: w721 -> [w725]
                tunnel: w720 -> [w730]
                tunnel: [w724] -> w718
                tunnel: w717 -> [w724]
                tunnel: [w738] -> w719
                tunnel: w718 -> [w738]
                tunnel: w719 -> [w740]
                frame #0 {
                  # "Iteration"
                  # "Error Info"
                  # "Last State"
                  # "Error Code"
                  # "Error Status"
                  n218 = Unbundle By Name(w733) -> ("status"=w732:bool, "code"=w727:i32)
                  n219 = Boolean To (0,1)(Boolean=w732) -> (0, 1=w731:i16)
                  n220 = To Long Integer(number=w731) -> (32bit integer=w729:i32)
                  n221 = case shown="3" w730 {
                    tunnel: [w734 w735 w736 w737] -> w728
                    tunnel: w729 -> [w734 _ _ _]
                    tunnel: w727 -> [_ w735 _ _]
                    tunnel: w726 -> [_ _ w736 _]
                    tunnel: w725 -> [_ _ _ w737]
                    frame Default {
                    }
                    frame 1 {
                    }
                    frame 2 {
                    }
                    frame 3 {
                    }
                  }
                  "Status" <- w728
                }
                frame #1 {
                  "Read Status Flag" <- TRUE ("Read Flag")
                }
                frame #2 {
                  n222 = call "Tick Count3"() -> ("Tick Count(mSec)"=w741:u32)
                  n223 = while {
                    tunnel: w741 -> [w747]
                    tunnel: w740 -> [w745]
                    stop <- w744 stop-if-true
                    n224 = call "Wait3"("Count(mSec)"=u32 1 ("Count(Ticks)")) -> ("Tick Count(mSec)"=w748:u32)
                    n225 = Subtract(x=w748, y=w747) -> (x-y=w746:u32)
                    n226 = Greater?(x=w746, y=w745) -> (0:w743:bool)
                    n227 = Compound Arithmetic op=OR(w743, "Ack Read Status") -> (w744:bool)
                  }
                }
                frame #3 {
                  n228 = local write "Ack Read Status"(FALSE ("Read Flag")) -> ()
                }
              }
            }
          }
          frame True {
            # "No Status from Cycle Mode"
          }
        }
        n229 = local write "Cmd"(WSVCAP_SHL_State."Idle" ("SPI_CMD_DBG")) -> ()
      }
    }
    n230 = Select(t=WSVCAP_SHL_Communication_Loop_State."Operation Complete" ("Action"), s=w19, f=w21) -> (s? t:f=w20:T3)
  }
  n231 = local write "Exit"(w4) -> ()
